vi "STED Control V2.vi"() -> ()   [LabVIEW 2014]
uses:
  FPGA-7842R-Reference.ctl
  Scan Parameters.ctl
  Manual Controls V2.ctl
  <vilib>/Utility/miscctls.llb/LVRectTypeDef.ctl
  <vilib>/Utility/miscctls.llb/LVPositionTypeDef.ctl
  Laser Controls.ctl
  XY_Stage/StageStates.ctl
  Type Defs/Image Acquisition Parameters.ctl
  Detectors.ctl
  Stage Control.ctl
panel:
  in  "Stage Control":T1={"Halt"=FALSE, "Home"=FALSE, "Down Stage"=FALSE, "Right Stage"=FALSE, "Up Stage"=FALSE, "Left Stage"=FALSE, "Mode"=enum."Joystick", "X Position"=1.0, "Y Position"=1.0, "Step Size (um)"=enum."2", "Velocity"=enum."Low"} {"Y Position" min=1.0 max=24.0}
  in  "Autoscale Z":bool
  in  "Reset Zoom":bool
  in  "Zoom Out":bool
  in  "Zoom In":bool
  in  "Pan":bool
  in  "Remove Display":bool
  in  "Add Display":bool
  in  "Colormap 2":u16(ring) items=["Fire", "Gray", "Red", "Green", "Blue", "Cyan", "Magenta", "Yellow", "Red-White", "Green-White", "Blue-White", "Glow"]
  in  "Merge Tool":bool
  in  "Smooth Tool":bool
  out "Channel 6":sgl[][](graph)
  out "Channel 5":sgl[][](graph)
  out "Channel 4":sgl[][](graph)
  out "Channel 3":sgl[][](graph)
  out "Channel 2":sgl[][](graph)
  in  "Dual Screens":bool=TRUE
  in  "Detectors":T2
  in  "Laser Controls":T3 {"590 Power (V)" scale=0.0..3.0; "STED Power (V)" scale=0.0..5.0}
  in  "Save File Path":path
  in  "Capture":bool
  in  "show cursor":bool
  in  "Set Mode Offset":bool
  in  "Unused Axis Voltage":i16=16300
  out "Channel 1":sgl[][](graph)
  in  "Image Acquisition Parameters":T4={"Scan Type"=enum."Sample Scanning", "Scan Mode"=enum."XY", "Fast Axis Frequency (Hz)"=100.0, "Image Format"=128, "Line Accumulations"=1, "Frames Per Capture"=1, "Frames Accumulations"=1, "Image Dimension (um)"=[], "Number of Z Steps"=1, "Z Steps Size (um)"=1.0, "Pixel Size (nm)"=[]} {"Z Steps Size (um)" min=0.0; "Number of Z Steps" min=1; "Frames Accumulations" min=1; "Frames Per Capture" min=1; "Line Accumulations" min=1; "Image Format" items=["64 x 64"=64, "128 x 128"=128, "256 x 256"=256, "512 x 512"=512, "1024 x 1024"=1024, "2048 x 2048"=2048]}
  in  "Live":bool
  in  "Exit":bool
  # "XY"
  # "Z"
  # "Length"
  # "Height"
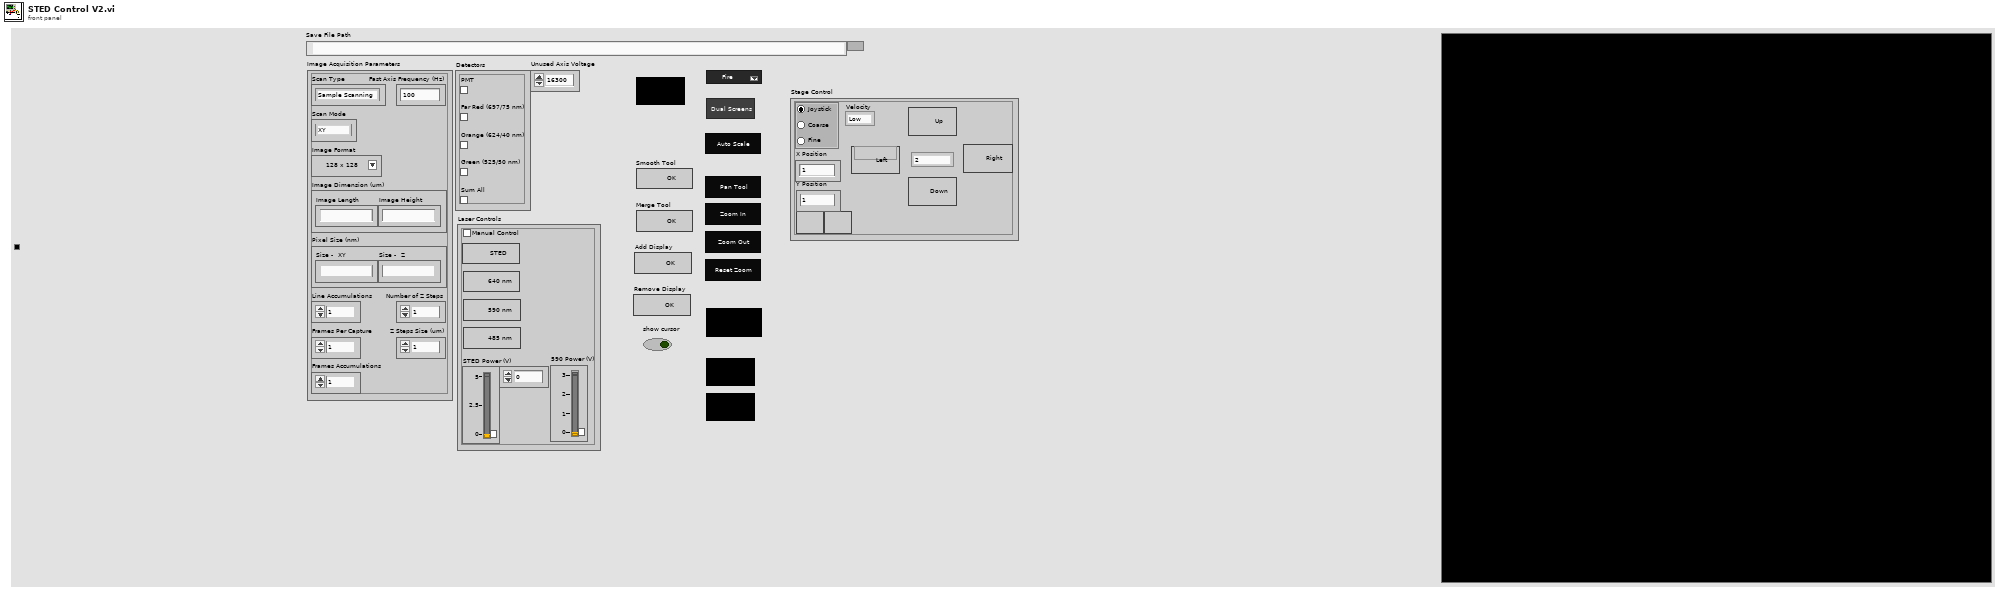
[diagram p1: front panel]
types:
  T1 = typedef "Stage Control.ctl" = cluster{"Halt":bool, "Home":bool, "Down Stage":bool, "Right Stage":bool, "Up Stage":bool, "Left Stage":bool, "Mode":enum32{"Joystick", "Coarse", "Fine"}, "X Position":dbl, "Y Position":dbl, "Step Size (um)":enum16{"1", "2", "5", "10", "15", "20", "50", "100", "500"}, "Velocity":enum16{"Low", "Medium", "High"}}
  T2 = typedef "Detectors.ctl" = cluster{"PMT":bool, "Far Red (697/75 nm)":bool, "Orange (624/40 nm)":bool, "Green (525/50 nm)":bool, "Sum All":bool}
  T3 = typedef "Laser Controls.ctl" = cluster{"STED Power (V)":dbl, "590 Power (V)":dbl, "STED":bool, "640 nm":bool, "590 nm":bool, "485 nm":bool, "Manual Control":bool}
  T4 = typedef "Image Acquisition Parameters.ctl" = cluster{"Scan Type":enum16{"Sample Scanning", "Beam Scanning"}, "Scan Mode":enum16{"XY", "XZ", "YZ", "XYZ"}, "Fast Axis Frequency (Hz)":dbl, "Image Format":u16, "Line Accumulations":u16, "Frames Per Capture":u16, "Frames Accumulations":u16, "Image Dimension (um)":dbl[], "Number of Z Steps":u8, "Z Steps Size (um)":dbl, "Pixel Size (nm)":dbl[]}
  T5 = typedef "Manual Controls V2.ctl" = cluster{"Galvo 1 Position (I16)":i16, "Galvo 2 Position (I16)":i16, "X Axis Voltage (I16)":i16, "Y Axis Voltage (I16)":i16, "Z Axis Voltage (I16)":i16, "Res Mirror Amp (I16)":i16, "Res Mirror Mute":bool}
  T6 = typedef "Scan Parameters.ctl" = cluster{"Fast_Ax_Amp_V":dbl, "Fast_Ax_Off_V":dbl, "Slow_Ax_Amp_V":dbl, "Slow_Ax_Off_V ":dbl, "Slow_Ax_Max_V_VperS":dbl, "Slow_Ax1_Del25ns":i32, "Slow_Ax2_Del25ns":i32, "Stage_X_Off_V":dbl, "Stage_Y_Off_V":dbl, "Stage_Z_Off_V":dbl, "Galvo1_Off_V":dbl, "Galvo2_Off_V":dbl, "Last_Scan_Mode":enum16{"XY", "XZ", "YZ", "XYZ"}, "Current_Scan_Mode":enum16{"XY", "XZ", "YZ", "XYZ"}, "Fly_Back_Lines":u16, "Linear_Ramp_End":u32, "Z_Step_I16":i16, "Z_Start_I16":i16, "Laser_States _U32":u32, "590_Voltage_I16":i16, "775_AOM_Volt_I16":i16, "Blanking OFF":bool, "Unused_Axis_I16":i16}
  T7 = typedef "FPGA-7842R-Reference.ctl" = enum16{"Stage Control", "Laser Control", "Unused Axis I16", "Exit", "Set Res Mirror", "Set Galvo", "Default", "Close FPGA", "Stop Waveforms", "Start Waveforms", "Initialize"}
  T8 = typedef "LVPositionTypeDef.ctl" = cluster{"Left":i32, "Top":i32}
  T9 = typedef "LVRectTypeDef.ctl" = cluster{"Left":i16, "Top":i16, "Right":i16, "Bottom":i16}
  T10 = enum32{"Invalid", "Standard", "Closed", "Hidden", "Minimized", "Maximized"}
  T11 = typedef "StageStates.ctl" = enum16{"POSITION", "MVR", "MOVE", "HALT", "ONTARGET", "ERROR", "EXIT", "HOME", "ZEROPOS", "NANOPOS", "QUIT", "SERVO", "JOYSTICK", "ANALOG"}
  T12 = typedef "LVRangeTypeDef.ctl" = cluster{"Minimum":dbl, "Maximum":dbl, "Increment":dbl, "Minor Increment":dbl, "Start":dbl}
  T13 = typedef "LVAllMonitorsDisplayTypeDef.ctl" = cluster{"Bounds":cluster{"Left":i16, "Top":i16, "Right":i16, "Bottom":i16}, "Depth":i16}[]
  T14 = cluster{"Bounds":cluster{"Left":i16, "Top":i16, "Right":i16, "Bottom":i16}, "Depth":i16}
  T15 = cluster{"Scan Type":bool, "Scan Mode":bool, "Fast Axis Frequency (Hz)":bool, "Image Format":bool, "Line Accumulations":bool, "Frames Per Capture":bool, "Frames Accumulations":bool, "Image Dimension (um)":bool[], "Number of Z Steps":bool, "Z Steps Size (um)":bool, "Pixel Size (nm)":bool[]}
  T16 = cluster{"Halt":bool, "Home":bool, "Down Stage":bool, "Right Stage":bool, "Up Stage":bool, "Left Stage":bool, "Mode":bool, "X Position":bool, "Y Position":bool, "Step Size (um)":bool, "Velocity":bool}
  T17 = enum16{"1", "2", "5", "10", "15", "20", "50", "100", "500"}
  T18 = typedef "Scanning Conversions.ctl" = cluster{"Stage X Axis (Volts/um)":dbl, "Stage Y Axis (Volts/um)":dbl, "Stage Z Axis (Volts/um)":dbl}
  T19 = typedef "IMAQ Image.ctl" = refnum<image>
  T20 = typedef "Waveform Data.ctl" = cluster{"Waveform Scan Parameters":cluster{"Scanning Mode":u8, "Fast Axis WF Length (Elements)":i32, "Fast Axis Sample Period (Ticks)":u32, "Slow Axis 1 WF Length (Elements)":i32, "Slow Axis 1 Sample Period (Ticks)":u32, "Slow Axis 1 Delay (25 ns) Steps":i32, "Slow Axis 2 WFLength (Elements)":i32, "Slow Axis 2 Sample Period (Ticks)":u32, "Slow Axis 2 Delay (25 ns) Steps":i32}, "Fast Axis Waveform":dbl[], "Slow Axis 1 Waveform":dbl[], "Slow Axis 2 Waveform":dbl[]}
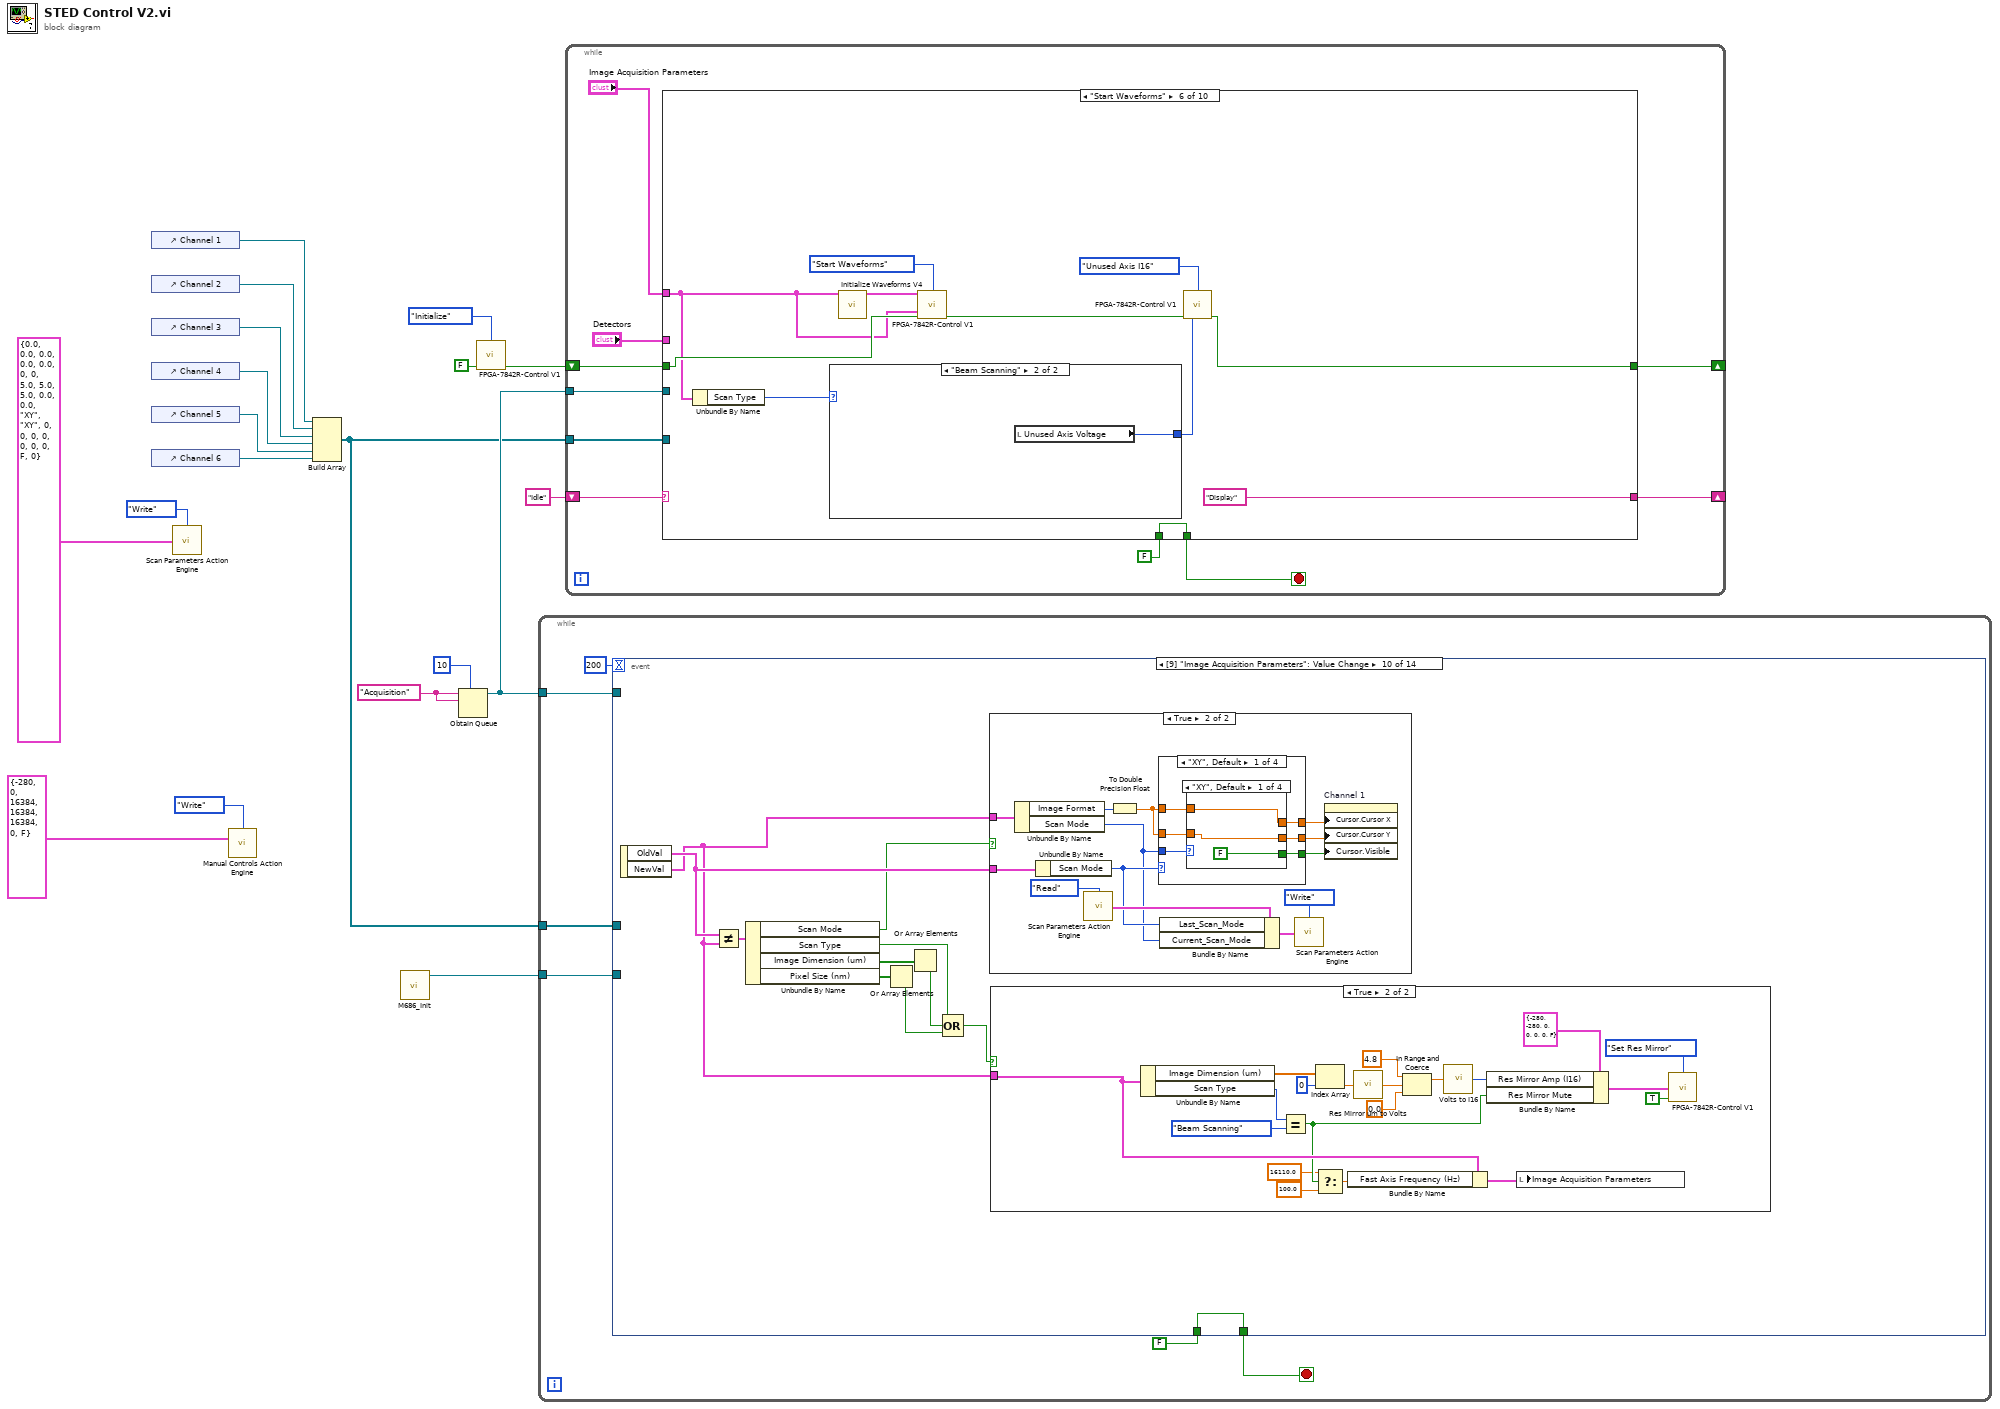
[diagram p0: block diagram]
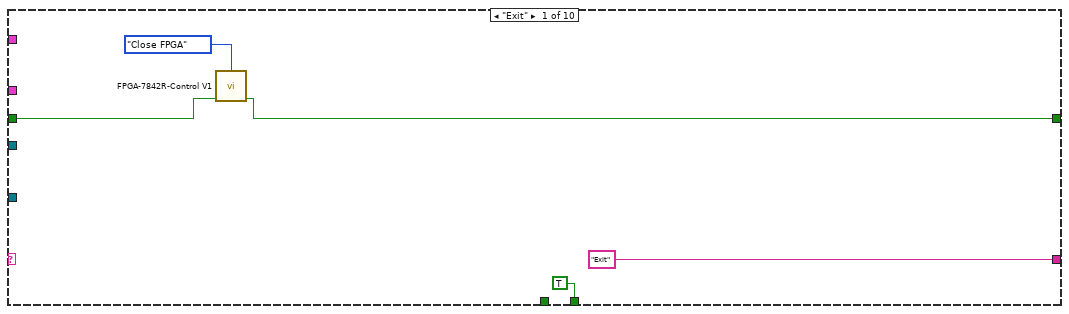
[diagram p2: hidden frame]
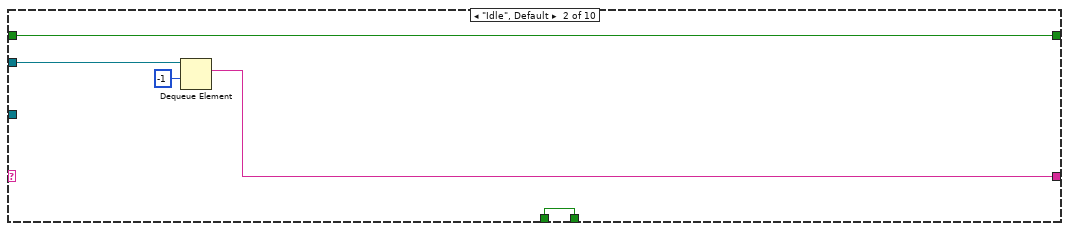
[diagram p3: hidden frame]
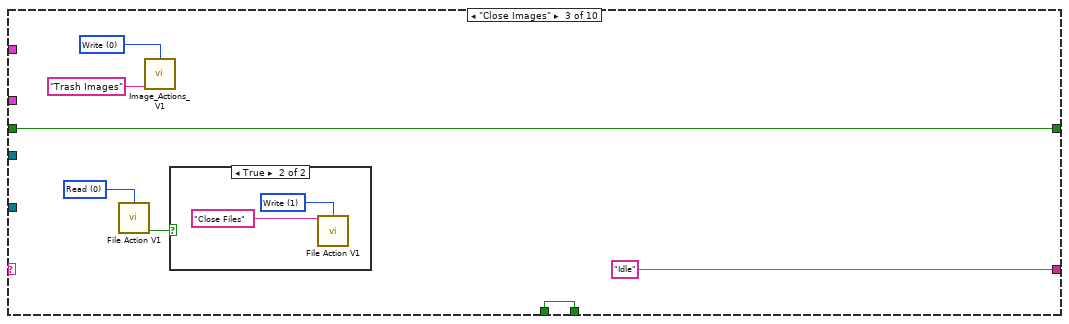
[diagram p4: hidden frame]
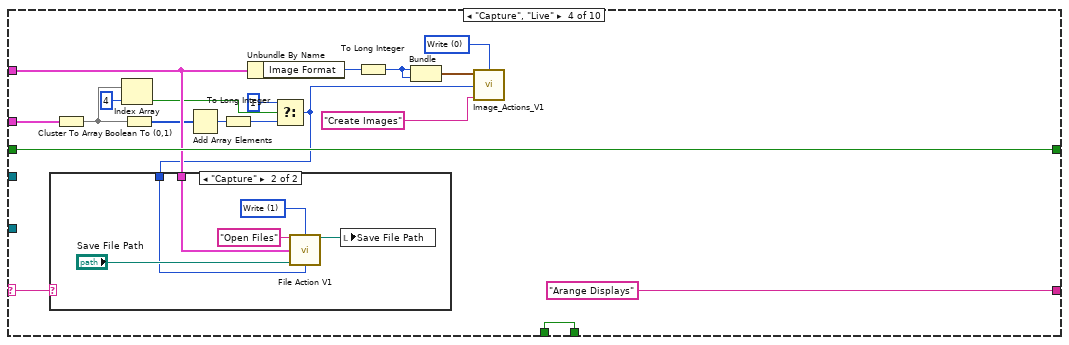
[diagram p6: hidden frame]
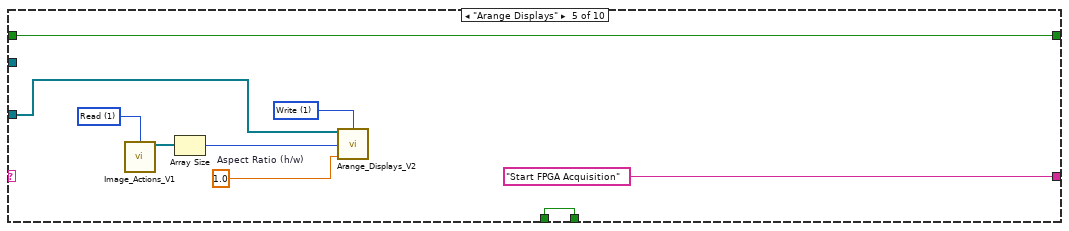
[diagram p8: hidden frame]
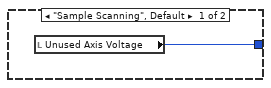
[diagram p9: hidden frame]
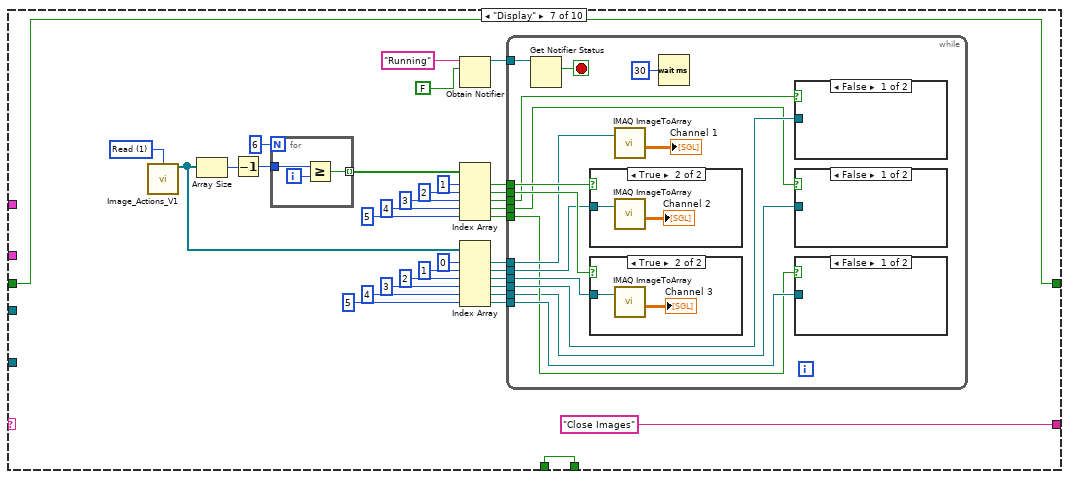
[diagram p10: hidden frame]
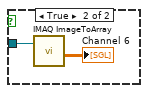
[diagram p11: hidden frame]
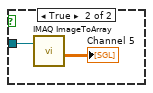
[diagram p12: hidden frame]
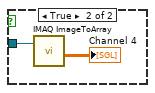
[diagram p13: hidden frame]
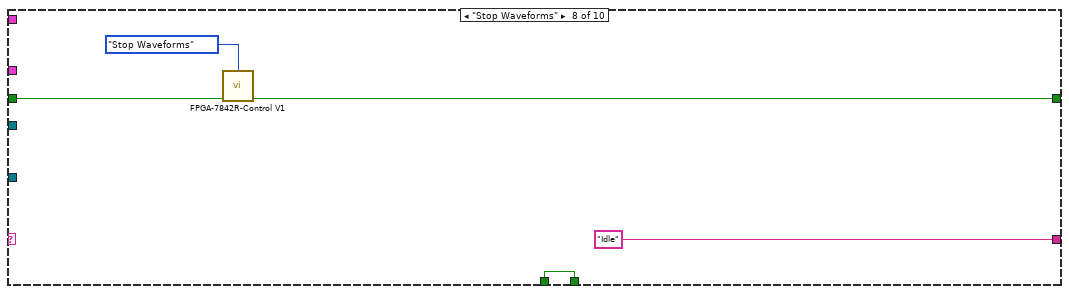
[diagram p16: hidden frame]
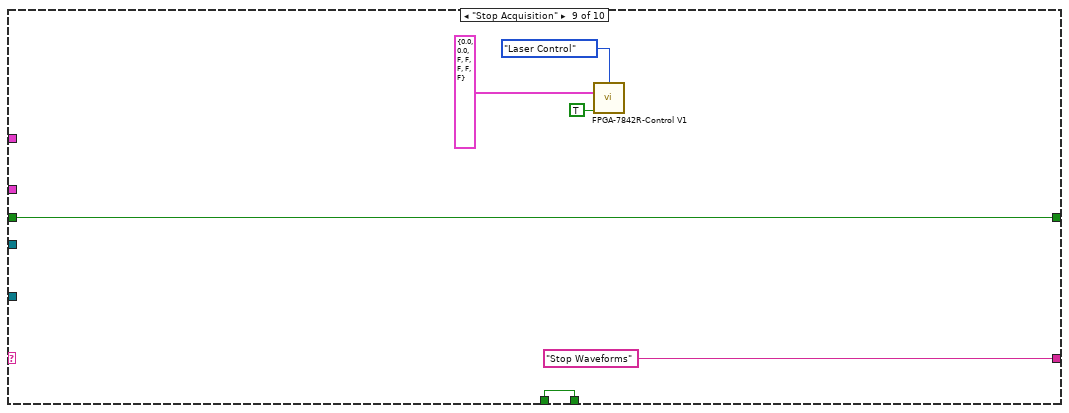
[diagram p17: hidden frame]
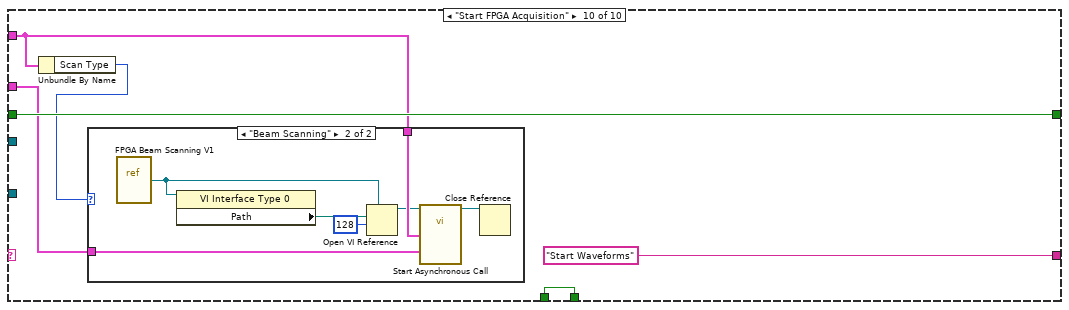
[diagram p18: hidden frame]
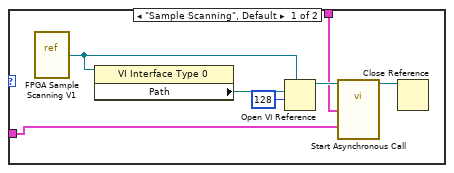
[diagram p19: hidden frame]
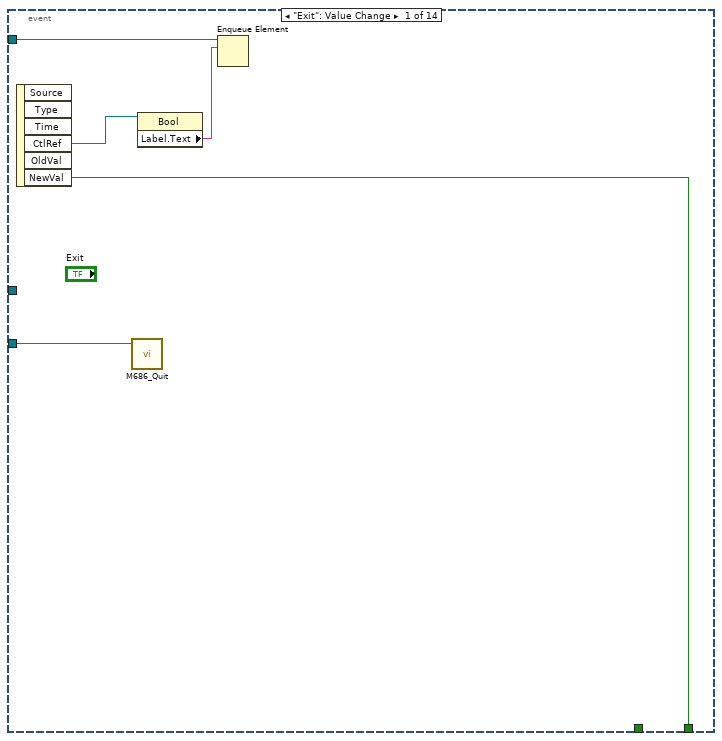
[diagram p20: hidden frame]
diagram:
  w18 = "Acquisition" ("name (unnamed)")
  n1 = control-ref of="Channel 1"() -> (w10:refnum<vi>)
  n2 = control-ref of="Channel 2"() -> (w9:refnum<vi>)
  n3 = control-ref of="Channel 3"() -> (w8:refnum<vi>)
  n4 = control-ref of="Channel 4"() -> (w7:refnum<vi>)
  n5 = control-ref of="Channel 5"() -> (w6:refnum<vi>)
  n6 = control-ref of="Channel 6"() -> (w5:refnum<vi>)
  n7 = call "Scan Parameters Action Engine.vi"("Action"=enum16{"Read", "Write"}."Write", "Scan Parameters IN"=T6 {"Fast_Ax_Amp_V"=0.0, "Fast_Ax_Off_V"=0.0, "Slow_Ax_Amp_V"=0.0, "Slow_Ax_Off_V "=0.0, "Slow_Ax_Max_V_VperS"=0.0, "Slow_Ax1_Del25ns"=0, "Slow_Ax2_Del25ns"=0, "Stage_X_Off_V"=5.0, "Stage_Y_Off_V"=5.0, "Stage_Z_Off_V"=5.0, "Galvo1_Off_V"=0.0, "Galvo2_Off_V"=0.0, "Last_Scan_Mode"=enum."XY", "Current_Scan_Mode"=enum."XY", "Fly_Back_Lines"=0, "Linear_Ramp_End"=0, "Z_Step_I16"=0, "Z_Start_I16"=0, "Laser_States _U32"=0, "590_Voltage_I16"=0, "775_AOM_Volt_I16"=0, "Blanking OFF"=FALSE, "Unused_Axis_I16"=0}) -> ()  [unwired: 13 in, 1 out]
  n8 = call "Manual Controls Action Engine.vi"("Action"=enum16{"Read", "Write"}."Write", "Manual Controls In"=T5 {"Galvo 1 Position (I16)"=-280, "Galvo 2 Position (I16)"=0, "X Axis Voltage (I16)"=16384, "Y Axis Voltage (I16)"=16384, "Z Axis Voltage (I16)"=16384, "Res Mirror Amp (I16)"=0, "Res Mirror Mute"=FALSE} ("Manual Controls")) -> ()  [unwired: 13 in, 1 out]
  n9 = Build Array(w10, w9, w8, w7, w6, w5) -> (w4:refnum<vi>[])
  n10 = call "M686_Init.vi"() -> ("VISA Refnum out"=w3:refnum<visa-resource-name>)  [unwired: 9 in, 2 out]
  n11 = Obtain Queue(max queue size (-1, unlimited)=10, name (unnamed)=w18, element data type=w18) -> (queue out=w16:refnum<queue>)  [unwired: 2 in, 2 out]
  n12 = call "FPGA-7842R-Control V1.vi"("Action"=FPGA-7842R-Reference."Initialize", "Initialize"=FALSE) -> ("Initalized"=w13:bool)  [unwired: 13 in]
  n13 = while {
    tunnel: w16 -> [w23]
    tunnel: w4 -> [w21]
    tunnel: w3 -> [w20]
    stop <- w25 stop-if-true
    n14 = event shown="[9] \"Image Acquisition Parameters\": Value Change" {
      selector: _ -> [_ _ _ _ _ _ _ _ _ _ _ _ _ _]
      dyn-events: _ -> [_ _ _ _ _ _ _ _ _ _ _ _ _ _]
      timeout: 200 -> [_ _ _ _ _ _ _ _ _ _ _ _ _ _]
      tunnel: [w30 w42 w47 w80 w107 w172 w192 w200 w227 w269 w419 w425 w611 w823] -> w25
      tunnel: FALSE -> [_ w42 w47 w80 w107 w172 w192 w200 w227 w269 w419 w425 w611 w823]
      tunnel: w23 -> [w29 w41 _ _ _ _ w186 _ _ _ _ _ _ _]
      tunnel: w21 -> [_ _ w44 _ w102 w171 _ _ _ _ _ _ _ _]
      tunnel: w20 -> [w26 _ _ _ _ _ _ _ _ _ _ w430 _ _]
      event "Exit": Value Change {
        n15 = event-data() -> ("CtlRef"=w28:refnum<vi>, "NewVal"=w30:bool)  [unwired: 1 in, 4 out]
        n16 = call "M686_Quit.vi"("VISA Refnum in"=w26) -> ()  [unwired: 11 in]
        n17 = property class="Bool"(reference=w28) -> ("Label.Text"=w27:string)  [unwired: 1 in, 2 out]
        n18 = Enqueue Element(queue=w29, element=w27) -> ()  [unwired: 2 in, 3 out]
      }
      event "Live", "Capture": Value Change {
        n19 = event-data() -> ("CtlRef"=w40:refnum<vi>, "NewVal"=w32:bool)  [unwired: 1 in]
        n20 = property on="Channel 1" class="IntGraph (strict)"("Cursor.Visible"=FALSE) -> ()  [unwired: 2 in, 2 out]
        n21 = property class="Bool (strict)"(reference=w40) -> ("Label.Text"=w31:string)  [unwired: 1 in, 2 out]
        n22 = Obtain Notifier(name (unnamed)="Running", notification data type=TRUE) -> (notifier out=w37:refnum<notifier>)  [unwired: 2 in, 2 out]
        n23 = Not(x=w32) -> (.not. x?=w35:bool)
        n24 = Send Notification(notification=w35, notifier=w37) -> ()  [unwired: 1 in, 2 out]
        n25 = Select(t=w31, s=w32, f="Stop Acquisition") -> (s? t:f=w33:string)
        n26 = Enqueue Element(queue=w41, element=w33) -> ()  [unwired: 2 in, 3 out]
      }
      event "Smooth Tool", "Merge Tool", "Add Display", "Remove Display", "Autoscale Z": Value Change {
        n27 = event-data() -> ("CtlRef"=w46:refnum<vi>)  [unwired: 1 in, 5 out]
        n28 = property class="Bool"(reference=w46) -> ("Label.Text"=w45:string)  [unwired: 1 in, 2 out]
        n29 = control-ref of="This VI"() -> (w43:refnum<vi>)
        n30 = case shown="\"Autoscale Z\"" w45 {
          tunnel: w44 -> [_ w49 w56 w61 w65 w71]
          tunnel: w43 -> [_ w48 _ _ _ w70]
          frame Default {
          }
          frame "Merge Tool" {
            n31 = vi-ref "MergeTool - Cambridge.vi"() -> (w53:refnum<vi>)
            n32 = property class="VI Interface Type 2"(reference=w53) -> ("Path"=w51:path)  [unwired: 1 in, 2 out]
            n33 = Open VI Reference(type specifier VI Refnum (for type only)=w53, vi path=w51, options=128) -> (vi reference=w52:refnum<vi>)  [unwired: 3 in, 1 out]
            n34 = call-by-ref "Start Asynchronous Call"(reference=w52, "VI Reference"=w48, "Display References"=w49) -> (reference out=w54:refnum<vi>)  [unwired: 11 in, 1 out]
            n35 = Close Reference(reference=w54) -> ()  [unwired: 1 in, 1 out]
          }
          frame "Add Display" {
            w59 = u16 1 items=["Read", "Write"] ("Action")
            w60 = u16 0 items=["Read", "Write"] ("Action")
            n36 = call "Arange_Displays_V2.vi"("Action"=w60) -> ("Number of Channels OUT"=w58:i32)  [unwired: 14 in]
            n37 = Increment(x=w58) -> (x+1=w57:i32)
            n38 = call "Arange_Displays_V2.vi"("Display References"=w56, "Action"=w59, "Number of Channels"=w57, "Aspect Ratio (h/w)"=1.0) -> ()  [unwired: 11 in, 1 out]
          }
          frame "Autoscale Z" {
            n39 = for {
              tunnel: w61 -> [w62] mode=indexing
              n40 = property class="IntGraph (strict)"(reference=w62, "ZScale.ScaleFit"=u8 1 ("Z Scale.Scale Fit")) -> ()  [unwired: 1 in, 2 out]
            }
          }
          frame "Remove Display" {
            w68 = u16 1 items=["Read", "Write"] ("Action")
            w69 = u16 0 items=["Read", "Write"] ("Action")
            n41 = call "Arange_Displays_V2.vi"("Action"=w69) -> ("Number of Channels OUT"=w67:i32)  [unwired: 14 in]
            n42 = Decrement(x=w67) -> (x-1=w66:i32)
            n43 = call "Arange_Displays_V2.vi"("Display References"=w65, "Action"=w68, "Number of Channels"=w66, "Aspect Ratio (h/w)"=1.0) -> ()  [unwired: 11 in, 1 out]
          }
          frame "Smooth Tool" {
            n44 = vi-ref "SmoothTool.vi"() -> (w73:refnum<vi>)
            n45 = property class="VI Interface Type 3"(reference=w73) -> ("Path"=w75:path)  [unwired: 1 in, 2 out]
            n46 = Open VI Reference(type specifier VI Refnum (for type only)=w73, vi path=w75, options=128) -> (vi reference=w74:refnum<vi>)  [unwired: 3 in, 1 out]
            n47 = call-by-ref "Start Asynchronous Call"(reference=w74, "VI Reference"=w70, "Display References"=w71) -> (reference out=w72:refnum<vi>)  [unwired: 2 in, 1 out]
            n48 = Close Reference(reference=w72) -> ()  [unwired: 1 in, 1 out]
          }
        }
      }
      event "Pan", "Zoom In", "Zoom Out", "Reset Zoom": Value Change {
        n49 = event-data() -> ("CtlRef"=w78:refnum<vi>, "NewVal"=w77:bool)  [unwired: 1 in]
        n50 = case shown="True" w77 {
          tunnel: w78 -> [_ w88]
          tunnel: [0 ("Palette:Active Tool") w87] -> w79
          frame False {
          }
          frame True {
            n51 = property class="Bool (strict)"(reference=w88) -> ("Label.Text"=w82:string)  [unwired: 1 in, 2 out]
            n52 = Build Array("Pan", "Zoom In", "Zoom Out") -> (w83:string[])
            n53 = case shown="\"Pan\"" w82 {
              tunnel: [6 ("Palette:Active Tool") 7 ("Palette:Active Tool") 5 ("Palette:Active Tool") 1 ("Palette:Active Tool")] -> w87
              frame "Zoom In" {
              }
              frame "Zoom Out" {
              }
              frame "Reset Zoom", Default {
              }
              frame "Pan" {
              }
            }
            n54 = for {
              tunnel: w83 -> [w89] mode=indexing
              tunnel: w82 -> [w93]
              n55 = Equal?(x=w93, y=w89) -> (x = y?=w90:bool)
              n56 = control-ref of="This VI"() -> (w91:refnum<vi>)
              n57 = To Variant(anything=w90) -> (Variant=w92:variant)
              n58 = invoke class="VI" method="Ctrl Val.Set"(reference=w91, "Control Name"=w89, "Value"=w92) -> ()  [unwired: 2 in, 5 out]
            }
          }
        }
        n59 = property on="Channel 1" class="IntGraph (strict)"("ActPaletteTool"=w79) -> ()  [unwired: 2 in, 2 out]
        n60 = property on="Channel 2" class="IntGraph (strict)"("ActPaletteTool"=w79) -> ()  [unwired: 2 in, 2 out]
        n61 = property on="Channel 3" class="IntGraph (strict)"("ActPaletteTool"=w79) -> ()  [unwired: 2 in, 2 out]
        n62 = property on="Channel 4" class="IntGraph (strict)"("ActPaletteTool"=w79) -> ()  [unwired: 2 in, 2 out]
        n63 = property on="Channel 5" class="IntGraph (strict)"("ActPaletteTool"=w79) -> ()  [unwired: 2 in, 2 out]
        n64 = property on="Channel 6" class="IntGraph (strict)"("ActPaletteTool"=w79) -> ()  [unwired: 2 in, 2 out]
      }
      event "Channel 1", "Channel 2", "Channel 3", "Channel 4", "Channel 5", "Channel 6": Mouse Down {
        n65 = event-data() -> ("CtlRef"=w103:refnum<vi>, "Mods.Double Click"=w106:bool, "PlatMods.Shift"=w105:bool, "PlatMods.Ctrl"=w104:bool)  [unwired: 1 in]
        n66 = Build Array(w106, w105, w104) -> (w99:bool[])
        n67 = property class="IntGraph (strict)"(reference=w103) -> (reference out=w101:refnum<vi>, "Label.Text"=w98:string)  [unwired: 1 in, 1 out]
        n68 = Boolean Array To Number(Boolean array=w99) -> (number=w100:u32)
        n69 = case shown="0" w100 {
          tunnel: w98 -> [w109 _ _ _ _]
          tunnel: w101 -> [_ w124 w159 w170 _]
          tunnel: w102 -> [w108 _ _ _ _]
          frame 0 {
            n70 = for {
              tunnel: w109 -> [w113]
              tunnel: w108 -> [w112] mode=indexing
              # "Single Click - Show Z Scale"
              n71 = property class="IntGraph (strict)"(reference=w112) -> (reference out=w110:refnum<vi>, "Label.Text"=w111:string)  [unwired: 1 in, 1 out]
              n72 = Equal?(x=w111, y=w113) -> (x = y?=w115:bool)
              n73 = Select(t=T8 {"Left"=2000, "Top"=17} ("Z Scale.Position"), s=w115, f=T8 {"Left"=0, "Top"=0} ("Z Scale.Position")) -> (s? t:f=w114:T8)
              n74 = property class="IntGraph (strict)"(reference=w110, "ZScale.Visible"=w115, "ZScale.Position"=w114) -> ()  [unwired: 1 in, 2 out]
            }
          }
          frame 2 {
            # "Shift Click - Apply color map."
            n75 = property class="IntGraph (strict)"(reference=w124) -> (reference out=w118:refnum<vi>, "ZScale.Maximum"=w119:dbl)  [unwired: 1 in, 1 out]
            n76 = case shown="0, Default" "Colormap 2" {
              tunnel: [cluster{dbl, u32}[] [{0.0, 0}, {85.0, 16711680}, {108.0, 16729344}, {127.0, 16744192}, {132.0, 16747520}, {140.0, 16753920}, {157.0, 16766720}, {170.0, 16776960}, {245.0, 16777184}, {250.0, 16777200}, {255.0, 16777215}] ("Z Scale.Marker Values[]") cluster{dbl, u32}[] [{0.0, 0}, {255.0, 16777215}] ("Z Scale.Marker Values[]") cluster{dbl, u32}[] [{0.0, 0}, {255.0, 16711680}] ("Z Scale.Marker Values[]") cluster{dbl, u32}[] [{0.0, 0}, {255.0, 65280}] ("Z Scale.Marker Values[]") cluster{dbl, u32}[] [{0.0, 0}, {255.0, 255}] ("Z Scale.Marker Values[]") cluster{dbl, u32}[] [{0.0, 0}, {255.0, 65535}] ("Z Scale.Marker Values[]") cluster{dbl, u32}[] [{0.0, 0}, {255.0, 16711935}] ("Z Scale.Marker Values[]") cluster{dbl, u32}[] [{0.0, 0}, {255.0, 16776960}] ("Z Scale.Marker Values[]") cluster{dbl, u32}[] [{0.0, 0}, {170.0, 16711680}, {245.0, 16777184}, {250.0, 16777200}, {255.0, 16448250}] ("Z Scale.Marker Values[]") cluster{dbl, u32}[] [{0.0, 0}, {170.0, 65280}, {245.0, 16777184}, {250.0, 16777200}, {255.0, 16448250}] ("Z Scale.Marker Values[]") cluster{dbl, u32}[] [{0.0, 0}, {170.0, 255}, {245.0, 16777184}, {250.0, 16777200}, {255.0, 16448250}] ("Z Scale.Marker Values[]") cluster{dbl, u32}[] [{0.0, 0}, {1.0, 131072}, {2.0, 196608}, {3.0, 327680}, {4.0, 458752}, {5.0, 589824}, {6.0, 720896}, {7.0, 851971}, {8.0, 983043}, {9.0, 1114115}, {10.0, 1245187}, {11.0, 1376259}, {12.0, 1507331}, {13.0, 1638403}, {14.0, 1769475}, {15.0, 1769479}, {16.0, 2031623}, {17.0, 2162695}, {18.0, 2293767}, {19.0, 2424839}, {20.0, 2555911}, {21.0, 2686983}, {22.0, 2818055}, {23.0, 2949127}, {24.0, 3080203}, {25.0, 3211275}, {26.0, 3342347}, {27.0, 3473419}, {28.0, 3604491}, {29.0, 3735563}, {30.0, 3866635}, {31.0, 3867403}, {32.0, 4129547}, {33.0, 4260619}, {34.0, 4391691}, {35.0, 4522763}, {36.0, 4653839}, {37.0, 4784911}, {38.0, 4915983}, {39.0, 5178127}, {40.0, 5309199}, {41.0, 5440271}, {42.0, 5571343}, {43.0, 5702415}, {44.0, 5703439}, {45.0, 5965583}, {46.0, 6096655}, {47.0, 6227727}, {48.0, 6358799}, {49.0, 6489871}, {50.0, 6620943}, {51.0, 6752015}, {52.0, 6883087}, {53.0, 7015183}, {54.0, 7146255}, {55.0, 7277327}, {56.0, 7408399}, {57.0, 7539471}, {58.0, 7670543}, {59.0, 7801615}, {60.0, 8063759}, {61.0, 8194831}, {62.0, 8326927}, {63.0, 8457999}, {64.0, 8589075}, {65.0, 8720147}, {66.0, 8851219}, {67.0, 8982291}, {68.0, 9113363}, {69.0, 9114387}, {70.0, 9376531}, {71.0, 9507603}, {72.0, 9638675}, {73.0, 9769747}, {74.0, 9901843}, {75.0, 10032915}, {76.0, 10163987}, {77.0, 10229523}, {78.0, 10295059}, {79.0, 10427155}, {80.0, 10558227}, {81.0, 10689299}, {82.0, 10820371}, {83.0, 10886931}, {84.0, 10952467}, {85.0, 11083539}, {86.0, 11214611}, {87.0, 11215635}, {88.0, 11477779}, {89.0, 11543315}, {90.0, 11608851}, {91.0, 11740947}, {92.0, 11806483}, {93.0, 11872019}, {94.0, 12004115}, {95.0, 12135187}, {96.0, 12266259}, {97.0, 12267283}, {98.0, 12398355}, {99.0, 12529427}, {100.0, 12530451}, {101.0, 12595987}, {102.0, 12530451}, {103.0, 12793619}, {104.0, 12794131}, {105.0, 12794643}, {106.0, 13056787}, {107.0, 13057299}, {108.0, 13057811}, {109.0, 13188883}, {110.0, 13320979}, {111.0, 13386515}, {112.0, 13452563}, {113.0, 13584147}, {114.0, 13584659}, {115.0, 13585171}, {116.0, 13585683}, {117.0, 13717267}, {118.0, 13848339}, {119.0, 13849363}, {120.0, 13849875}, {121.0, 13850387}, {122.0, 13981459}, {123.0, 14113555}, {124.0, 14114067}, {125.0, 14114579}, {126.0, 14115091}, {127.0, 14246675}, {128.0, 14377747}, {129.0, 14378771}, {130.0, 14379283}, {131.0, 14379539}, {132.0, 14379795}, {133.0, 14380819}, {134.0, 14511891}, {135.0, 14643987}, {136.0, 14644503}, {137.0, 14645015}, {138.0, 14645527}, {139.0, 14646039}, {140.0, 14646551}, {141.0, 14778135}, {142.0, 14909207}, {143.0, 14910231}, {144.0, 14910747}, {145.0, 14911259}, {146.0, 14911771}, {147.0, 14912283}, {148.0, 14912797}, {149.0, 15044383}, {150.0, 15175455}, {151.0, 15175967}, {152.0, 15176479}, {153.0, 15176991}, {154.0, 15177507}, {155.0, 15178019}, {156.0, 15178531}, {157.0, 15310115}, {158.0, 15441701}, {159.0, 15441959}, {160.0, 15442215}, {161.0, 15442727}, {162.0, 15443243}, {163.0, 15443755}, {164.0, 15444269}, {165.0, 15444783}, {166.0, 15444783}, {167.0, 15576367}, {168.0, 15707953}, {169.0, 15708467}, {170.0, 15708979}, {171.0, 15708981}, {172.0, 15708983}, {173.0, 15710011}, {174.0, 15710523}, {175.0, 15711037}, {176.0, 15711039}, {177.0, 15711553}, {178.0, 15843139}, {179.0, 15974213}, {180.0, 15974215}, {181.0, 15974217}, {182.0, 15974219}, {183.0, 15975755}, {184.0, 15976271}, {185.0, 15976785}, {186.0, 15977299}, {187.0, 15977301}, {188.0, 15977815}, {189.0, 15978327}, {190.0, 15978331}, {191.0, 16109917}, {192.0, 16241503}, {193.0, 16241505}, {194.0, 16242019}, {195.0, 16242535}, {196.0, 16242537}, {197.0, 16242539}, {198.0, 16243563}, {199.0, 16243567}, {200.0, 16244081}, {201.0, 16244595}, {202.0, 16244599}, {203.0, 16244601}, {204.0, 16244603}, {205.0, 16245627}, {206.0, 16245631}, {207.0, 16245633}, {208.0, 16246147}, {209.0, 16246663}, {210.0, 16377735}, {211.0, 16508811}, {212.0, 16508815}, {213.0, 16509839}, {214.0, 16509843}, {215.0, 16509845}, {216.0, 16509847}, {217.0, 16510361}, {218.0, 16510875}, {219.0, 16510879}, {220.0, 16510881}, {221.0, 16510883}, {222.0, 16511399}, {223.0, 16511911}, {224.0, 16511915}, {225.0, 16511917}, {226.0, 16511919}, {227.0, 16511923}, {228.0, 16512437}, {229.0, 16512951}, {230.0, 16512955}, {231.0, 16512957}, {232.0, 16512959}, {233.0, 16512961}, {234.0, 16512963}, {235.0, 16512967}, {236.0, 16513481}, {237.0, 16513995}, {238.0, 16513999}, {239.0, 16514001}, {240.0, 16514003}, {241.0, 16514005}, {242.0, 16514007}, {243.0, 16514011}, {244.0, 16514013}, {245.0, 16514015}, {246.0, 16514019}, {247.0, 16514021}, {248.0, 16514023}, {249.0, 16514027}, {250.0, 16514029}, {251.0, 16514031}, {252.0, 16514035}, {253.0, 16514037}, {254.0, 16514039}, {255.0, 16514043}] ("Z Scale.Marker Values[]")] -> w122
              tunnel: w119 -> [w125 w127 w129 w131 w133 w135 w137 w139 w141 w143 w145 w148]
              tunnel: [w125 w127 w129 w131 w133 w135 w137 w139 w141 w143 w145 w148] -> w123
              frame 0, Default {
                # "Fire"
              }
              frame 1 {
                # "Grayscale"
              }
              frame 2 {
                # "Red"
              }
              frame 3 {
                # "Green"
              }
              frame 4 {
                # "Blue"
              }
              frame 5 {
                # "Cyan"
              }
              frame 6 {
                # "Magenta"
              }
              frame 7 {
                # "Yellow"
              }
              frame 8 {
                # "Red-White"
              }
              frame 9 {
                # "Green-White"
              }
              frame 10 {
                # "Blue-White"
              }
              frame 11 {
              }
            }
            n77 = property class="IntGraph (strict)"(reference=w118, "ZScale.MarkerVals[]"=w122, "ZScale.High Color"=u32 255, "ZScale.Maximum"=w123) -> ()  [unwired: 1 in, 2 out]
          }
          frame 6 {
            w158 = u16 1 items=["Get Image", "Load and Read File"] ("Action")
            # "Shift Control Click - Open Image"
            n78 = call "OpenDBL.vi"("Action"=w158) -> ("Image"=w157:sgl[], "Dimensions (Z, Y, X, t)"=w156:i32[])  [unwired: 12 in, 1 out]
            n79 = Index Array(array=w156, index #1=1 ("index"), index #2=2 ("index")) -> (element #1=w153:i32, element #2=w151:i32)
            n80 = Reverse 1D Array(array=w157) -> (reversed array=w150:sgl[])
            n81 = Reshape Array(w150, w153, w151) -> (w152:sgl[][])
            n82 = Transpose 2D Array(2D array=w152) -> (transposed array=w149:sgl[][])
            n83 = property class="IntGraph (strict)"(reference=w159, "Value"=w149) -> ()  [unwired: 1 in, 2 out]
          }
          frame 4 {
            # "Control Click - Open for feature fitting"
            n84 = property class="IntGraph (strict)"(reference=w170) -> ("Value"=w164:sgl[][])  [unwired: 1 in, 2 out]
            n85 = local read "Image Acquisition Parameters"() -> (w163:T4)
            n86 = vi-ref "QuickProfile_V3.vi"() -> (w169:refnum<vi>)
            n87 = property class="VI Interface Type 5"(reference=w169) -> ("Path"=w166:path)  [unwired: 1 in, 2 out]
            n88 = Unbundle By Name(w163) -> ("Pixel Size (nm)"=w162:dbl[])
            n89 = Index Array(array=w162, index=0) -> (element=w160:dbl)
            n90 = Open VI Reference(type specifier VI Refnum (for type only)=w169, vi path=w166, options=128) -> (vi reference=w168:refnum<vi>)  [unwired: 3 in, 1 out]
            n91 = call-by-ref "Start Asynchronous Call"(reference=w168, "Image IN"=w164, "Pixel Size (nm)"=w160) -> (reference out=w165:refnum<vi>)  [unwired: 15 in, 1 out]
            n92 = Close Reference(reference=w165) -> ()  [unwired: 1 in, 1 out]
          }
          frame 10, Default {
            # "No match case"
          }
        }
      }
      event "Channel 1", "Channel 2", "Channel 3", "Channel 4", "Channel 5", "Channel 6": Mouse Up {
        n93 = event-data() -> ("CtlRef"=w173:refnum<vi>)  [unwired: 1 in]
        n94 = property class="IntGraph (strict)"(reference=w173) -> (reference out=w174:refnum<vi>, "ActPaletteTool"=w177:i32)  [unwired: 1 in, 1 out]
        n95 = Not Equal?(x=w177, y=0) -> (x != y?=w175:bool)
        n96 = case shown="True" w175 {
          tunnel: w174 -> [_ w181]
          tunnel: w171 -> [_ w178]
          frame False {
          }
          frame True {
            n97 = property class="IntGraph (strict)"(reference=w181) -> ("XScale.Range"=w180:T12, "YScale.Range"=w179:T12)  [unwired: 1 in, 2 out]
            n98 = for {
              tunnel: w180 -> [w183]
              tunnel: w179 -> [w184]
              tunnel: w178 -> [w182] mode=indexing
              n99 = property class="IntGraph (strict)"(reference=w182, "XScale.Range"=w183, "YScale.Range"=w184) -> ()  [unwired: 1 in, 2 out]
            }
          }
        }
      }
      event Timeout {
        n100 = event-data() -> ()  [unwired: 1 in, 3 out]
        n101 = Obtain Notifier(name (unnamed)="Running", notification data type=TRUE) -> (notifier out=w190:refnum<notifier>)  [unwired: 2 in, 2 out]
        n102 = Get Notifier Status(notifier=w190) -> (current notification=w188:bool)  [unwired: 1 in, 4 out]
        n103 = local read "Capture"() -> (w187:bool)
        n104 = And(x=w188, y=w187) -> (x .and. y?=w185:bool)
        n105 = case shown="False" w185 {
          tunnel: w186 -> [_ w194]
          frame False {
          }
          frame True {
            n106 = local write "Capture"(FALSE ("Capture")) -> ()
            n107 = Enqueue Element(queue=w194, element="Stop Acquisition" ("f")) -> ()  [unwired: 2 in, 3 out]
          }
        }
      }
      event Value Change {
        w213 = FALSE ("element")
        n108 = event-data() -> ()  [unwired: 1 in, 6 out]
        n109 = Unbundle By Name("Laser Controls") -> ("STED"=w219:bool, "640 nm"=w216:bool, "590 nm"=w217:bool, "485 nm"=w218:bool, "590 Power (V)"=w210:dbl, "STED Power (V)"=w209:dbl, "Manual Control"=w197:bool)
        n110 = Build Array(w219, w216, w217, w218, w213, w213, w213, w213) -> (w215:bool[])
        n111 = local read "Live"() -> (w198:bool)
        n112 = Boolean Array To Number(Boolean array=w215) -> (number=w214:u32)
        n113 = To Unsigned Byte Integer(number=w214) -> (unsigned 8bit integer=w212:u8)
        n114 = Or(x=w198, y=w197) -> (x .or. y?=w196:bool)
        n115 = call "U8_To_U32.vi"("U8 IN"=w212) -> ("U32 OUT"=w211:u32)  [unwired: 13 in, 1 out]
        n116 = case shown="True" w196 {
          tunnel: "Laser Controls" -> [_ w225]
          frame False {
          }
          frame True {
            n117 = call "FPGA-7842R-Control V1.vi"("Action"=FPGA-7842R-Reference."Laser Control", "Laser Controls"=w225, "Initialize"=TRUE) -> ()  [unwired: 12 in, 1 out]
          }
        }
        n118 = In Range and Coerce(upper limit=3.0, x=w210, lower limit=0.0) -> (coerced(x)=w204:dbl)  [unwired: 1 out]
        n119 = In Range and Coerce(upper limit=5.0, x=w209, lower limit=0.0) -> (coerced(x)=w203:dbl)  [unwired: 1 out]
        n120 = call "Volts to I16.vi"("Voltage (V)"=w204) -> ("I16"=w202:i16)  [unwired: 13 in, 1 out]
        n121 = call "Volts to I16.vi"("Voltage (V)"=w203) -> ("I16"=w201:i16)  [unwired: 13 in, 1 out]
        n122 = call "Scan Parameters Action Engine.vi"("Action"=enum16{"Read", "Write"}."Read") -> ("Scan Parameters OUT"=w222:T6)  [unwired: 14 in]
        n123 = Bundle By Name(cluster=w222, "Laser_States _U32"=w211, "590_Voltage_I16"=w202, "775_AOM_Volt_I16"=w201) -> (w220:T6)
        n124 = call "Scan Parameters Action Engine.vi"("Action"=enum16{"Read", "Write"}."Write", "Scan Parameters IN"=w220) -> ()  [unwired: 13 in, 1 out]
      }
      event "Dual Screens": Value Change {
        n125 = event-data() -> ("NewVal"=w229:bool)  [unwired: 1 in, 5 out]
        n126 = property class="App"() -> ("Disp.AllMonitors"=w230:T13)  [unwired: 2 in, 2 out]
        n127 = control-ref of="This VI"() -> (w228:refnum<vi>)
        n128 = case shown="False" w229 {
          tunnel: w230 -> [w233 w246]
          tunnel: T9 {"Left"=0, "Top"=0, "Right"=0, "Bottom"=0} ("FP Window Bounds 2") -> [w232 w245]
          tunnel: w228 -> [_ w244]
          frame False {
            w236 = i16 0
            n129 = Index Array(array=w233, index=0) -> (element=w240:T14)
            n130 = Unbundle By Name(w240) -> ("Bounds.Right"=w241:i16, "Bounds.Bottom"=w238:i16, "Bounds.Top"=w237:i16)
            n131 = Subtract(x=w238, y=w237) -> (x-y=w235:i16)
            n132 = Bundle By Name(cluster=w232, "Left"=w236, "Top"=w236, "Right"=w241, "Bottom"=w235) -> (w234:T9)
            n133 = property class="VI"("Front Panel.WinBounds"=w234) -> (reference out=w243:refnum<vi>)  [unwired: 2 in, 1 out]
            n134 = property class="VI"(reference=w243, "FP.State"=T10."Maximized" ("Front Panel Window:State")) -> ()  [unwired: 1 in, 2 out]
          }
          frame True {
            w255 = i16 0
            n135 = Index Array(array=w246, index #1=1 ("index"), index #2=0 ("index")) -> (element #1=w249:T14, element #2=w250:T14)
            n136 = Unbundle By Name(w249) -> ("Bounds.Right"=w251:i16)
            n137 = Unbundle By Name(w250) -> ("Bounds.Left"=w252:i16, "Bounds.Bottom"=w253:i16, "Bounds.Top"=w254:i16)
            n138 = Subtract(x=w251, y=w252) -> (x-y=w256:i16)
            n139 = Subtract(x=w253, y=w254) -> (x-y=w257:i16)
            n140 = Bundle By Name(cluster=w245, "Left"=w255, "Top"=w255, "Right"=w256, "Bottom"=w257) -> (w258:T9)
            n141 = property class="VI"(reference=w244, "Front Panel.WinBounds"=w258) -> ()  [unwired: 1 in, 2 out]
          }
        }
      }
      event Value Change {
        n142 = event-data() -> ("OldVal"=w268:T4, "NewVal"=w265:T4)  [unwired: 1 in]
        n143 = Not Equal?(x=w268, y=w265) -> (x != y?=w267:T15)
        n144 = Unbundle By Name(w267) -> ("Scan Mode"=w266:bool, "Scan Type"=w264:bool, "Image Dimension (um)"=w263:bool[], "Pixel Size (nm)"=w262:bool[])
        n145 = Or Array Elements(Boolean array=w262) -> (logical OR=w259:bool)
        n146 = Or Array Elements(Boolean array=w263) -> (logical OR=w260:bool)
        n147 = Compound Arithmetic op=OR(w264, w260, w259) -> (w261:bool)
        n148 = case shown="True" w266 {
          tunnel: w265 -> [_ w292]
          tunnel: w268 -> [_ w302]
          frame False {
            n149 = property on="Channel 1" class="IntGraph (strict)"("Cursor.Visible"=FALSE) -> ()  [unwired: 2 in, 2 out]
          }
          frame True {
            n150 = Unbundle By Name(w292) -> ("Image Format"=w303:u16, "Scan Mode"=w295:enum16{"XY", "XZ", "YZ", "XYZ"})
            n151 = Unbundle By Name(w302) -> ("Scan Mode"=w296:enum16{"XY", "XZ", "YZ", "XYZ"})
            n152 = call "Scan Parameters Action Engine.vi"("Action"=enum16{"Read", "Write"}."Read") -> ("Scan Parameters OUT"=w298:T6)  [unwired: 14 in]
            n153 = To Double Precision Float(number=w303) -> (double precision float=w291:dbl)
            n154 = case shown="\"XY\", Default" w296 {
              tunnel: w291 -> [w308 w336 w364 w392]
              tunnel: w291 -> [w307 w335 w363 w391]
              tunnel: w295 -> [w309 w337 w365 w393]
              tunnel: [w306 w334 w362 w390] -> w301
              tunnel: [w305 w333 w361 w389] -> w300
              tunnel: [w304 w332 w360 w388] -> w299
              frame "XY", Default {
                n155 = case shown="\"XY\", Default" w309 {
                  tunnel: w308 -> [w311 w318 w323 w325]
                  tunnel: w307 -> [w312 w315 w322 w329]
                  tunnel: [w311 w314 w320 w326] -> w306
                  tunnel: [w312 w313 w319 w330] -> w305
                  tunnel: [FALSE ("Cursor.Visible") TRUE ("Cursor.Visible") TRUE ("Cursor.Visible") FALSE ("Cursor.Visible")] -> w304
                  frame "XY", Default {
                  }
                  frame "XZ" {
                    n156 = Divide(x=w318, y=2.0) -> (x/y=w313:dbl)
                    n157 = Increment(x=w315) -> (x+1=w314:dbl)
                  }
                  frame "YZ" {
                    n158 = Increment(x=w323) -> (x+1=w319:dbl)
                    n159 = Divide(x=w322, y=2.0) -> (x/y=w320:dbl)
                  }
                  frame "XYZ" {
                    n160 = Divide(x=w325, y=2.0) -> (x/y=w326:dbl)
                    n161 = Divide(x=w329, y=2.0) -> (x/y=w330:dbl)
                  }
                }
              }
              frame "XZ" {
                n162 = case shown="\"XY\"" w337 {
                  tunnel: w336 -> [w339 w346 w350 w353]
                  tunnel: w335 -> [w341 w345 w348 w357]
                  tunnel: [w338 w346 w347 w354] -> w334
                  tunnel: [w340 w345 w349 w358] -> w333
                  tunnel: [TRUE ("Cursor.Visible") FALSE ("Cursor.Visible") TRUE ("Cursor.Visible") FALSE ("Cursor.Visible")] -> w332
                  frame "XY" {
                    n163 = Increment(x=w339) -> (x+1=w338:dbl)
                    n164 = Divide(x=w341, y=2.0) -> (x/y=w340:dbl)
                  }
                  frame "XZ", Default {
                  }
                  frame "YZ" {
                    n165 = Divide(x=w350, y=2.0) -> (x/y=w347:dbl)
                    n166 = Increment(x=w348) -> (x+1=w349:dbl)
                  }
                  frame "XYZ" {
                    n167 = Divide(x=w353, y=2.0) -> (x/y=w354:dbl)
                    n168 = Divide(x=w357, y=2.0) -> (x/y=w358:dbl)
                  }
                }
              }
              frame "YZ" {
                n169 = case shown="\"XYZ\"" w365 {
                  tunnel: w364 -> [w367 w375 w378 w386]
                  tunnel: w363 -> [w369 w373 w382 w387]
                  tunnel: [w366 w372 w379 w386] -> w362
                  tunnel: [w368 w374 w383 w387] -> w361
                  tunnel: [TRUE ("Cursor.Visible") TRUE ("Cursor.Visible") FALSE ("Cursor.Visible") FALSE ("Cursor.Visible")] -> w360
                  frame "XY" {
                    n170 = Increment(x=w367) -> (x+1=w366:dbl)
                    n171 = Divide(x=w369, y=2.0) -> (x/y=w368:dbl)
                  }
                  frame "XZ" {
                    n172 = Divide(x=w375, y=2.0) -> (x/y=w372:dbl)
                    n173 = Increment(x=w373) -> (x+1=w374:dbl)
                  }
                  frame "XYZ" {
                    n174 = Divide(x=w378, y=2.0) -> (x/y=w379:dbl)
                    n175 = Divide(x=w382, y=2.0) -> (x/y=w383:dbl)
                  }
                  frame "YZ", Default {
                  }
                }
              }
              frame "XYZ" {
                n176 = case shown="\"YZ\"" w393 {
                  tunnel: w392 -> [w394 w406 w411 w414]
                  tunnel: w391 -> [w398 w401 w408 w415]
                  tunnel: [w395 w405 w410 w414] -> w390
                  tunnel: [w399 w402 w409 w415] -> w389
                  tunnel: [FALSE ("Cursor.Visible") TRUE ("Cursor.Visible") TRUE ("Cursor.Visible") FALSE ("Cursor.Visible")] -> w388
                  frame "XY" {
                    n177 = Divide(x=w394, y=2.0) -> (x/y=w395:dbl)
                    n178 = Divide(x=w398, y=2.0) -> (x/y=w399:dbl)
                  }
                  frame "XZ" {
                    n179 = Divide(x=w406, y=2.0) -> (x/y=w405:dbl)
                    n180 = Increment(x=w401) -> (x+1=w402:dbl)
                  }
                  frame "YZ" {
                    n181 = Increment(x=w411) -> (x+1=w410:dbl)
                    n182 = Divide(x=w408, y=2.0) -> (x/y=w409:dbl)
                  }
                  frame "XYZ", Default {
                  }
                }
              }
            }
            n183 = Bundle By Name(cluster=w298, "Last_Scan_Mode"=w296, "Current_Scan_Mode"=w295) -> (w293:T6)
            n184 = call "Scan Parameters Action Engine.vi"("Action"=enum16{"Read", "Write"}."Write", "Scan Parameters IN"=w293) -> ()  [unwired: 13 in, 1 out]
            n185 = property on="Channel 1" class="IntGraph (strict)"("Cursor.Cursor X"=w301, "Cursor.Cursor Y"=w300, "Cursor.Visible"=w299) -> ()  [unwired: 2 in, 2 out]
          }
        }
        n186 = case shown="True" w261 {
          tunnel: w265 -> [_ w275]
          frame False {
          }
          frame True {
            n187 = Unbundle By Name(w275) -> ("Image Dimension (um)"=w289:dbl[], "Scan Type"=w284:enum16{"Sample Scanning", "Beam Scanning"})
            n188 = Equal?(x=w284, y=enum16{"Sample Scanning", "Beam Scanning"}."Beam Scanning") -> (x = y?=w274:bool)
            n189 = Index Array(array=w289, index=0) -> (element=w282:dbl)
            n190 = Select(t=16110.0, s=w274, f=100.0) -> (s? t:f=w271:dbl)
            n191 = Bundle By Name(cluster=w275, "Fast Axis Frequency (Hz)"=w271) -> (w270:T4)
            n192 = call "Res Mirror um to Volts.vi"("Image Size (um)"=w282) -> ("Voltage (V)"=w281:dbl)
            n193 = In Range and Coerce(upper limit=4.8, x=w281, lower limit=0.0) -> (coerced(x)=w280:dbl)  [unwired: 1 out]
            n194 = call "Volts to I16.vi"("Voltage (V)"=w280) -> ("I16"=w285:i16)  [unwired: 13 in, 1 out]
            n195 = Bundle By Name(cluster=T5 {"Galvo 1 Position (I16)"=-280, "Galvo 2 Position (I16)"=-280, "X Axis Voltage (I16)"=0, "Y Axis Voltage (I16)"=0, "Z Axis Voltage (I16)"=0, "Res Mirror Amp (I16)"=0, "Res Mirror Mute"=FALSE} ("Manual Controls"), "Res Mirror Amp (I16)"=w285, "Res Mirror Mute"=w274) -> (w276:T5)
            n196 = local write "Image Acquisition Parameters"(w270) -> ()
            n197 = call "FPGA-7842R-Control V1.vi"("Action"=FPGA-7842R-Reference."Set Res Mirror", "Manual Controls"=w276, "Initialize"=TRUE) -> ()  [unwired: 12 in, 1 out]
          }
        }
      }
      event "Unused Axis Voltage": Value Change {
        n198 = event-data() -> ()  [unwired: 1 in, 6 out]
        n199 = call "FPGA-7842R-Control V1.vi"("Action"=FPGA-7842R-Reference."Unused Axis I16", "Initialize"=TRUE, "Unused Axis Offset (I16)"="Unused Axis Voltage") -> ()  [unwired: 12 in, 1 out]
      }
      event Value Change {
        n200 = event-data() -> ("OldVal"=w436:T1, "NewVal"=w429:T1)  [unwired: 1 in, 4 out]
        n201 = Not Equal?(x=w436, y=w429) -> (x != y?=w435:T16)
        n202 = property on="Stage Control" class="Clust"() -> ("Controls[]"=w434:refnum<vi>[])  [unwired: 2 in, 2 out]
        n203 = Cluster To Array(cluster=w435) -> (array=w433:bool[])
        n204 = for {
          tunnel: w434 -> [w608] mode=indexing
          tunnel: w433 -> [w609] mode=indexing
          tunnel: [w608] -> w432
          stop <- w609 stop-if-true
        }
        n205 = Unbundle By Name(w429) -> ("Step Size (um)"=w426:T17, "Mode"=w431:enum32{"Joystick", "Coarse", "Fine"})
        n206 = property class="Ctl"(reference=w432) -> ("ClassName"=w428:string, "Label.Text"=w427:string)  [unwired: 1 in, 2 out]
        n207 = control-ref of="Halt"() -> (w420:refnum<vi>)
        n208 = case shown="\"Fine\"" w431 {
          tunnel: w430 -> [w443 w455 w527 w538]
          tunnel: w428 -> [_ w454 _ w537]
          tunnel: w427 -> [_ w453 _ w536]
          tunnel: w426 -> [_ w447 _ w533]
          tunnel: "Stage Control" -> [_ _ _ _]
          tunnel: [w438 w446 w526 w530] -> w423
          tunnel: w420 -> [w437 w445 w525 w529]
          frame "Joystick" {
            w442 = TRUE
            n209 = Build Array(w442, w442) -> (w441:bool[])
            n210 = call "M686.vi"("Abort"=w437, "Axis"=w441, "Action"=StageStates."JOYSTICK", "VISA In"=w443) -> ("VISA Out"=w440:refnum<visa-resource-name>)  [unwired: 4 in, 3 out]
            n211 = call "M686.vi"("Abort"=w437, "Action"=StageStates."POSITION", "VISA In"=w440) -> ("Position Out"=w438:dbl[])  [unwired: 5 in, 3 out]
          }
          frame "Coarse" {
            w457 = FALSE
            n212 = Build Array(w457, w457) -> (w456:bool[])
            n213 = Format Into String(w447) -> (resulting string=w451:string)  [unwired: 3 in, 1 out]
            n214 = call "M686.vi"("Abort"=w445, "Axis"=w456, "Action"=StageStates."JOYSTICK", "VISA In"=w455) -> ("VISA Out"=w452:refnum<visa-resource-name>)  [unwired: 4 in, 3 out]
            n215 = Fract/Exp String To Number(string=w451) -> (number=w450:dbl)  [unwired: 3 in, 1 out]
            n216 = Divide(x=w450, y=1000.0) -> (x/y=w449:dbl)
            n217 = case shown="\"Boolean\"" w454 {
              tunnel: w453 -> [_ w467]
              tunnel: w452 -> [w462 w466]
              tunnel: w449 -> [_ w465]
              tunnel: w445 -> [w459 w464]
              tunnel: [w461 w463] -> w446
              frame Default {
                n218 = call "M686.vi"("Abort"=w459, "Action"=StageStates."POSITION", "VISA In"=w462) -> ("Position Out"=w461:dbl[])  [unwired: 5 in, 3 out]
              }
              frame "Boolean" {
                n219 = case shown="\"Right\"" w467 {
                  tunnel: w466 -> [_ w472 w479 w492 w503 w514 w524]
                  tunnel: w465 -> [_ _ _ w489 w500 w511 w517]
                  tunnel: w464 -> [_ w470 w477 w484 w494 w505 w516]
                  tunnel: [dbl[] [] ("Position Out") w469 w476 w483 w493 w504 w515] -> w463
                  frame Default {
                  }
                  frame "Home" {
                    w474 = TRUE
                    n220 = Build Array(w474, w474) -> (w475:bool[])
                    n221 = call "M686.vi"("Velocity"=1.0, "Abort"=w470, "Axis"=w475, "Action"=StageStates."HOME", "VISA In"=w472) -> ("Position Out"=w469:dbl[])  [unwired: 3 in, 3 out]
                  }
                  frame "Halt" {
                    w481 = TRUE
                    n222 = Build Array(w481, w481) -> (w482:bool[])
                    n223 = call "M686.vi"("Velocity"=1.0, "Abort"=w477, "Axis"=w482, "Action"=StageStates."HALT", "VISA In"=w479) -> ("Position Out"=w476:dbl[])  [unwired: 3 in, 3 out]
                  }
                  frame "Up" {
                    n224 = Build Array(w489, w489) -> (w488:dbl[])
                    n225 = Build Array(FALSE, TRUE) -> (w485:bool[])
                    n226 = call "M686.vi"("Velocity"=1.0, "Abort"=w484, "Axis"=w485, "Positions"=w488, "Action"=StageStates."MVR", "VISA In"=w492) -> ("Position Out"=w483:dbl[])  [unwired: 2 in, 3 out]
                  }
                  frame "Down" {
                    n227 = Negate(x=w500) -> (-x=w495:dbl)
                    n228 = Build Array(w495, w495) -> (w499:dbl[])
                    n229 = Build Array(FALSE, TRUE) -> (w496:bool[])
                    n230 = call "M686.vi"("Velocity"=1.0, "Abort"=w494, "Axis"=w496, "Positions"=w499, "Action"=StageStates."MVR", "VISA In"=w503) -> ("Position Out"=w493:dbl[])  [unwired: 2 in, 3 out]
                  }
                  frame "Left" {
                    n231 = Negate(x=w511) -> (-x=w506:dbl)
                    n232 = Build Array(w506, w506) -> (w510:dbl[])
                    n233 = Build Array(TRUE, FALSE) -> (w507:bool[])
                    n234 = call "M686.vi"("Velocity"=1.0, "Abort"=w505, "Axis"=w507, "Positions"=w510, "Action"=StageStates."MVR", "VISA In"=w514) -> ("Position Out"=w504:dbl[])  [unwired: 2 in, 3 out]
                  }
                  frame "Right" {
                    n235 = Build Array(w517, w517) -> (w521:dbl[])
                    n236 = Build Array(TRUE, FALSE) -> (w518:bool[])
                    n237 = call "M686.vi"("Velocity"=1.0, "Abort"=w516, "Axis"=w518, "Positions"=w521, "Action"=StageStates."MVR", "VISA In"=w524) -> ("Position Out"=w515:dbl[])  [unwired: 2 in, 3 out]
                  }
                }
              }
            }
          }
          frame Default {
            n238 = call "M686.vi"("Abort"=w525, "Action"=StageStates."POSITION", "VISA In"=w527) -> ("Position Out"=w526:dbl[])  [unwired: 5 in, 3 out]
          }
          frame "Fine" {
            w540 = FALSE
            n239 = Build Array(w540, w540) -> (w539:bool[])
            n240 = call "M686.vi"("Abort"=w529, "Axis"=w539, "Action"=StageStates."JOYSTICK", "VISA In"=w538) -> ("VISA Out"=w532:refnum<visa-resource-name>)  [unwired: 4 in, 3 out]
            n241 = Format Into String(w533) -> (resulting string=w535:string)  [unwired: 3 in, 1 out]
            n242 = call "M686.vi"("Abort"=w529, "Action"=StageStates."POSITION", "VISA In"=w532) -> ("Position Out"=w530:dbl[])  [unwired: 5 in, 3 out]
            n243 = Fract/Exp String To Number(string=w535) -> (number=w534:dbl)  [unwired: 3 in, 1 out]
            n244 = case shown="\"Boolean\"" w537 {
              tunnel: w536 -> [_ w555]
              tunnel: w534 -> [_ w554]
              frame "False", Default {
              }
              frame "Boolean" {
                n245 = call "Manual Controls Action Engine.vi"("Action"=enum16{"Read", "Write"}."Read") -> ("Manual Controls Out"=w547:T5)  [unwired: 14 in]
                n246 = call "Scan Parameters Action Engine.vi"("Action"=enum16{"Read", "Write"}."Read") -> ("Scan Parameters OUT"=w551:T6)  [unwired: 14 in]
                n247 = call "Scanning Volts to Microns.vi"() -> ("Scanning Conversions OUT"=w553:T18)
                n248 = case shown="\"Down\"" w555 {
                  tunnel: w554 -> [_ w566 _ w583 w594 w605]
                  tunnel: w553 -> [_ w568 _ w585 w596 w607]
                  tunnel: w551 -> [w557 w563 w574 w580 w591 w602]
                  tunnel: [w557 w562 w573 w579 w590 w601] -> w549
                  tunnel: w547 -> [w556 w560 w572 w577 w588 w599]
                  tunnel: [w556 w558 w571 w575 w586 w597] -> w545
                  frame Default {
                  }
                  frame "Up" {
                    n249 = Unbundle By Name(w568) -> ("Stage Y Axis (Volts/um)"=w567:dbl)
                    n250 = Unbundle By Name(w563) -> ("Stage_Y_Off_V"=w565:dbl)
                    n251 = Multiply(x=w566, y=w567) -> (x*y=w564:dbl)
                    n252 = Add(x=w565, y=w564) -> (x+y=w561:dbl)
                    n253 = call "Volts to I16.vi"("Voltage (V)"=w561) -> ("I16"=w559:i16)  [unwired: 13 in, 1 out]
                    n254 = Bundle By Name(cluster=w563, "Stage_Y_Off_V"=w561) -> (w562:T6)
                    n255 = Bundle By Name(cluster=w560, "Y Axis Voltage (I16)"=w559) -> (w558:T5)
                  }
                  frame "Home" {
                    w570 = 5.0 ("Stage Y Axis Offset (V)")
                    n256 = call "Volts to I16.vi"("Voltage (V)"=w570) -> ("I16"=w569:i16)  [unwired: 13 in, 1 out]
                    n257 = Bundle By Name(cluster=w574, "Stage_X_Off_V"=w570, "Stage_Y_Off_V"=w570, "Stage_Z_Off_V"=w570) -> (w573:T6)
                    n258 = Bundle By Name(cluster=w572, "X Axis Voltage (I16)"=w569, "Y Axis Voltage (I16)"=w569, "Z Axis Voltage (I16)"=w569) -> (w571:T5)
                  }
                  frame "Down" {
                    n259 = Unbundle By Name(w585) -> ("Stage Y Axis (Volts/um)"=w584:dbl)
                    n260 = Unbundle By Name(w580) -> ("Stage_Y_Off_V"=w582:dbl)
                    n261 = Multiply(x=w583, y=w584) -> (x*y=w581:dbl)
                    n262 = Subtract(x=w582, y=w581) -> (x-y=w578:dbl)
                    n263 = call "Volts to I16.vi"("Voltage (V)"=w578) -> ("I16"=w576:i16)  [unwired: 13 in, 1 out]
                    n264 = Bundle By Name(cluster=w580, "Stage_Y_Off_V"=w578) -> (w579:T6)
                    n265 = Bundle By Name(cluster=w577, "Y Axis Voltage (I16)"=w576) -> (w575:T5)
                  }
                  frame "Left" {
                    n266 = Unbundle By Name(w596) -> ("Stage X Axis (Volts/um)"=w595:dbl)
                    n267 = Unbundle By Name(w591) -> ("Stage_X_Off_V"=w593:dbl)
                    n268 = Multiply(x=w594, y=w595) -> (x*y=w592:dbl)
                    n269 = Subtract(x=w593, y=w592) -> (x-y=w589:dbl)
                    n270 = call "Volts to I16.vi"("Voltage (V)"=w589) -> ("I16"=w587:i16)  [unwired: 13 in, 1 out]
                    n271 = Bundle By Name(cluster=w591, "Stage_X_Off_V"=w589) -> (w590:T6)
                    n272 = Bundle By Name(cluster=w588, "X Axis Voltage (I16)"=w587) -> (w586:T5)
                  }
                  frame "Right" {
                    n273 = Unbundle By Name(w607) -> ("Stage X Axis (Volts/um)"=w606:dbl)
                    n274 = Unbundle By Name(w602) -> ("Stage_X_Off_V"=w604:dbl)
                    n275 = Multiply(x=w605, y=w606) -> (x*y=w603:dbl)
                    n276 = Add(x=w604, y=w603) -> (x+y=w600:dbl)
                    n277 = call "Volts to I16.vi"("Voltage (V)"=w600) -> ("I16"=w598:i16)  [unwired: 13 in, 1 out]
                    n278 = Bundle By Name(cluster=w602, "Stage_X_Off_V"=w600) -> (w601:T6)
                    n279 = Bundle By Name(cluster=w599, "X Axis Voltage (I16)"=w598) -> (w597:T5)
                  }
                }
                n280 = call "Manual Controls Action Engine.vi"("Action"=enum16{"Read", "Write"}."Write", "Manual Controls In"=w545) -> ("Manual Controls Out"=w544:T5)  [unwired: 13 in]
                n281 = call "Scan Parameters Action Engine.vi"("Action"=enum16{"Read", "Write"}."Write", "Scan Parameters IN"=w549) -> ()  [unwired: 13 in, 1 out]
                n282 = call "FPGA-7842R-Control V1.vi"("Action"=FPGA-7842R-Reference."Stage Control", "Manual Controls"=w544, "Initialize"=TRUE) -> ()  [unwired: 12 in, 1 out]
              }
            }
          }
        }
        n283 = Index Array(array=w423) -> (element #1=w422:dbl, element #2=w421:dbl)  [unwired: 2 in]
        n284 = property on="X Position" class="DigNum (strict)"("Value"=w422) -> ()  [unwired: 2 in, 2 out]
        n285 = property on="Y Position" class="DigNum (strict)"("Value"=w421) -> ()  [unwired: 2 in, 2 out]
      }
      event "Set Mode Offset": Value Change {
        n286 = event-data() -> ("NewVal"=w610:bool)  [unwired: 1 in]
        n287 = case shown="True" w610 {
          frame False {
          }
          frame True {
            # "Vert Pixels"
            # "Horz Pixels"
            # "Z Pixel Size"
            # "XY Pixel Size"
            # "Z volts per um"
            # "XY volts per um"
            n288 = local read "Image Acquisition Parameters"() -> (w625:T4)
            n289 = Unbundle By Name(w625) -> ("Image Format"=w626:u16, "Image Dimension (um)"=w629:dbl[])
            n290 = call "Scanning Volts to Microns.vi"() -> ("Scanning Conversions OUT"=w614:T18)
            n291 = Unbundle By Name(w614) -> ("Stage X Axis (Volts/um)"=w613:dbl, "Stage Z Axis (Volts/um)"=w612:dbl)
            n292 = property on="Channel 1" class="IntGraph (strict)"() -> ("Cursor.Cursor X"=w620:dbl, "Cursor.Cursor Y"=w621:dbl)  [unwired: 2 in, 2 out]
            n293 = To Double Precision Float(number=w626) -> (double precision float=w617:dbl)
            n294 = call "Scan Parameters Action Engine.vi"("Action"=enum16{"Read", "Write"}."Read") -> ("Scan Parameters OUT"=w634:T6)  [unwired: 14 in]
            n295 = Divide(x=w629, y=w617) -> (x/y=w630:dbl[])
            n296 = Unbundle By Name(w634) -> ("Last_Scan_Mode"=w623:enum16{"XY", "XZ", "YZ", "XYZ"}, "Current_Scan_Mode"=w624:enum16{"XY", "XZ", "YZ", "XYZ"})
            n297 = Index Array(array=w630, index #1=0 ("index"), index #2=1 ("index")) -> (element #1=w631:dbl, element #2=w632:dbl)
            n298 = Divide(x=w617, y=2.0) -> (x/y=w616:dbl)
            n299 = case shown="\"XY\", Default" w623 {
              tunnel: w624 -> [w639 w702 w749 w796]
              tunnel: w620 -> [w640 w694 w741 w788]
              tunnel: w621 -> [w641 w695 w742 w789]
              tunnel: w616 -> [w647 w701 w748 w795]
              tunnel: w631 -> [w646 w700 w747 w794]
              tunnel: w612 -> [w644 w698 w745 w792]
              tunnel: w613 -> [w645 w699 w746 w793]
              tunnel: w632 -> [w643 w697 w744 w791]
              tunnel: w616 -> [w642 w696 w743 w790]
              tunnel: w634 -> [w638 w693 w740 w787]
              tunnel: [w637 w692 w739 w786] -> w635
              tunnel: [w636 w691 w738 w785] -> w619
              frame "XY", Default {
                # "XY Scan Mode"
                n300 = case shown="\"YZ\"" w639 {
                  tunnel: w647 -> [w656 _ w682 _]
                  tunnel: w646 -> [w658 w676 w687 _]
                  tunnel: w645 -> [w657 w674 w685 _]
                  tunnel: w644 -> [_ _ _ _]
                  tunnel: w643 -> [_ _ _ _]
                  tunnel: w642 -> [w654 w672 _ _]
                  tunnel: w641 -> [w655 w671 _ _]
                  tunnel: w640 -> [w663 _ w681 _]
                  tunnel: w638 -> [w662 w668 w680 w690]
                  tunnel: [w661 w669 w679 w690] -> w637
                  tunnel: [w666 w667 w678 w689] -> w636
                  frame "XY", Default {
                    # "XY - No change"
                    n301 = Unbundle By Name(w662) -> ("Stage_X_Off_V"=w652:dbl, "Stage_Y_Off_V"=w650:dbl, "Stage_Z_Off_V"=w666:dbl)
                    n302 = Subtract(x=w663, y=w656) -> (x-y=w665:dbl)
                    n303 = Multiply(x=w665, y=w658) -> (x*y=w664:dbl)
                    n304 = Multiply(x=w664, y=w657) -> (x*y=w653:dbl)
                    n305 = Subtract(x=w655, y=w654) -> (x-y=w659:dbl)
                    n306 = Multiply(x=w659, y=w658) -> (x*y=w660:dbl)
                    n307 = Add(x=w652, y=w653) -> (x+y=w651:dbl)
                    n308 = Multiply(x=w660, y=w657) -> (x*y=w649:dbl)
                    n309 = Add(x=w650, y=w649) -> (x+y=w648:dbl)
                    n310 = Bundle By Name(cluster=w662, "Stage_X_Off_V"=w651, "Stage_Y_Off_V"=w648) -> (w661:T6)
                  }
                  frame "XZ" {
                    # "XZ - Grab Y cusor position - Set Y offset"
                    n311 = Subtract(x=w671, y=w672) -> (x-y=w677:dbl)
                    n312 = Unbundle By Name(w668) -> ("Stage_Y_Off_V"=w670:dbl)
                    n313 = Multiply(x=w677, y=w676) -> (x*y=w675:dbl)
                    n314 = Multiply(x=w675, y=w674) -> (x*y=w673:dbl)
                    n315 = Add(x=w670, y=w673) -> (x+y=w667:dbl)
                    n316 = Bundle By Name(cluster=w668, "Stage_Y_Off_V"=w667) -> (w669:T6)
                  }
                  frame "YZ" {
                    # "YZ - Grab X cursor position - Set X offset"
                    n317 = Subtract(x=w681, y=w682) -> (x-y=w688:dbl)
                    n318 = Unbundle By Name(w680) -> ("Stage_X_Off_V"=w684:dbl)
                    n319 = Multiply(x=w688, y=w687) -> (x*y=w686:dbl)
                    n320 = Multiply(x=w686, y=w685) -> (x*y=w683:dbl)
                    n321 = Add(x=w684, y=w683) -> (x+y=w678:dbl)
                    n322 = Bundle By Name(cluster=w680, "Stage_X_Off_V"=w678) -> (w679:T6)
                  }
                  frame "XYZ" {
                    # "XYZ - No change"
                    n323 = Unbundle By Name(w690) -> ("Stage_Z_Off_V"=w689:dbl)
                  }
                }
              }
              frame "XZ" {
                # "XZ Scan Mode"
                n324 = case shown="\"YZ\"" w702 {
                  tunnel: w701 -> [_ _ w718 _]
                  tunnel: w700 -> [_ _ w725 _]
                  tunnel: w699 -> [_ _ w722 _]
                  tunnel: w698 -> [w705 _ _ w729]
                  tunnel: w693 -> [w712 w715 w724 w736]
                  tunnel: w697 -> [w704 _ _ w728]
                  tunnel: [w709 w715 w719 w733] -> w692
                  tunnel: w696 -> [w708 _ _ w732]
                  tunnel: w695 -> [w707 _ _ w731]
                  tunnel: w694 -> [_ _ w717 _]
                  tunnel: [w703 w714 w716 w727] -> w691
                  frame "XY", Default {
                    # "XY - Grab Y cusor position - Set Z offset"
                    n325 = Subtract(x=w707, y=w708) -> (x-y=w713:dbl)
                    n326 = Unbundle By Name(w712) -> ("Stage_Z_Off_V"=w706:dbl)
                    n327 = Multiply(x=w713, y=w704) -> (x*y=w711:dbl)
                    n328 = Multiply(x=w711, y=w705) -> (x*y=w710:dbl)
                    n329 = Add(x=w706, y=w710) -> (x+y=w703:dbl)
                    n330 = Bundle By Name(cluster=w712, "Stage_Z_Off_V"=w703) -> (w709:T6)
                  }
                  frame "XZ" {
                    # "XZ - No change"
                    n331 = Unbundle By Name(w715) -> ("Stage_Z_Off_V"=w714:dbl)
                  }
                  frame "YZ" {
                    # "YZ - Grab X cursor position - Set X offset"
                    n332 = Subtract(x=w717, y=w718) -> (x-y=w726:dbl)
                    n333 = Unbundle By Name(w724) -> ("Stage_X_Off_V"=w721:dbl)
                    n334 = Multiply(x=w726, y=w725) -> (x*y=w723:dbl)
                    n335 = Multiply(x=w723, y=w722) -> (x*y=w720:dbl)
                    n336 = Add(x=w721, y=w720) -> (x+y=w716:dbl)
                    n337 = Bundle By Name(cluster=w724, "Stage_X_Off_V"=w716) -> (w719:T6)
                  }
                  frame "XYZ" {
                    # "XYZ - Grab Y cusor position - Set Z offset"
                    n338 = Subtract(x=w731, y=w732) -> (x-y=w737:dbl)
                    n339 = Unbundle By Name(w736) -> ("Stage_Z_Off_V"=w730:dbl)
                    n340 = Multiply(x=w737, y=w728) -> (x*y=w735:dbl)
                    n341 = Multiply(x=w735, y=w729) -> (x*y=w734:dbl)
                    n342 = Add(x=w730, y=w734) -> (x+y=w727:dbl)
                    n343 = Bundle By Name(cluster=w736, "Stage_Z_Off_V"=w727) -> (w733:T6)
                  }
                }
              }
              frame "YZ" {
                # "YZ Scan Mode"
                n344 = case shown="\"XZ\"" w749 {
                  tunnel: w748 -> [_ w763 _ _]
                  tunnel: w747 -> [_ w770 _ _]
                  tunnel: w746 -> [_ w767 _ _]
                  tunnel: w745 -> [w752 _ _ w776]
                  tunnel: w740 -> [w759 w769 w773 w783]
                  tunnel: w744 -> [w751 _ _ w775]
                  tunnel: [w756 w764 w773 w780] -> w739
                  tunnel: w743 -> [w755 _ _ w779]
                  tunnel: w742 -> [w754 _ _ w778]
                  tunnel: w741 -> [_ w762 _ _]
                  tunnel: [w750 w761 w772 w774] -> w738
                  frame "XY", Default {
                    # "XY - Grab Y cusor position - Set Z offset"
                    n345 = Subtract(x=w754, y=w755) -> (x-y=w760:dbl)
                    n346 = Unbundle By Name(w759) -> ("Stage_Z_Off_V"=w753:dbl)
                    n347 = Multiply(x=w760, y=w751) -> (x*y=w758:dbl)
                    n348 = Multiply(x=w758, y=w752) -> (x*y=w757:dbl)
                    n349 = Add(x=w753, y=w757) -> (x+y=w750:dbl)
                    n350 = Bundle By Name(cluster=w759, "Stage_Z_Off_V"=w750) -> (w756:T6)
                  }
                  frame "XZ" {
                    # "XZ - Grab X cursor position - Set Y offset"
                    n351 = Subtract(x=w762, y=w763) -> (x-y=w771:dbl)
                    n352 = Unbundle By Name(w769) -> ("Stage_Y_Off_V"=w766:dbl)
                    n353 = Multiply(x=w771, y=w770) -> (x*y=w768:dbl)
                    n354 = Multiply(x=w768, y=w767) -> (x*y=w765:dbl)
                    n355 = Add(x=w766, y=w765) -> (x+y=w761:dbl)
                    n356 = Bundle By Name(cluster=w769, "Stage_Y_Off_V"=w761) -> (w764:T6)
                  }
                  frame "YZ" {
                    # "YZ - No change"
                    n357 = Unbundle By Name(w773) -> ("Stage_Z_Off_V"=w772:dbl)
                  }
                  frame "XYZ" {
                    # "XYZ - Grab Y cusor position - Set Z offset"
                    n358 = Subtract(x=w778, y=w779) -> (x-y=w784:dbl)
                    n359 = Unbundle By Name(w783) -> ("Stage_Z_Off_V"=w777:dbl)
                    n360 = Multiply(x=w784, y=w775) -> (x*y=w782:dbl)
                    n361 = Multiply(x=w782, y=w776) -> (x*y=w781:dbl)
                    n362 = Add(x=w777, y=w781) -> (x+y=w774:dbl)
                    n363 = Bundle By Name(cluster=w783, "Stage_Z_Off_V"=w774) -> (w780:T6)
                  }
                }
              }
              frame "XYZ" {
                # "XYZ Scan Mode"
                n364 = case shown="\"XZ\"" w796 {
                  tunnel: w795 -> [_ _ w812 _]
                  tunnel: w794 -> [_ w808 w819 _]
                  tunnel: w793 -> [_ w805 w816 _]
                  tunnel: w792 -> [_ _ _ _]
                  tunnel: w787 -> [w798 w807 w818 w822]
                  tunnel: w791 -> [_ _ _ _]
                  tunnel: [w798 w803 w813 w822] -> w786
                  tunnel: w790 -> [_ w802 _ _]
                  tunnel: w789 -> [_ w801 _ _]
                  tunnel: w788 -> [_ _ w811 _]
                  tunnel: [w797 w799 w810 w821] -> w785
                  frame "XY", Default {
                    # "XY - No change"
                    n365 = Unbundle By Name(w798) -> ("Stage_Z_Off_V"=w797:dbl)
                  }
                  frame "XZ" {
                    # "XZ - Grab Y cusor position - Set Y offset"
                    n366 = Subtract(x=w801, y=w802) -> (x-y=w809:dbl)
                    n367 = Unbundle By Name(w807) -> ("Stage_Y_Off_V"=w800:dbl)
                    n368 = Multiply(x=w809, y=w808) -> (x*y=w806:dbl)
                    n369 = Multiply(x=w806, y=w805) -> (x*y=w804:dbl)
                    n370 = Add(x=w800, y=w804) -> (x+y=w799:dbl)
                    n371 = Bundle By Name(cluster=w807, "Stage_Y_Off_V"=w799) -> (w803:T6)
                  }
                  frame "YZ" {
                    # "YZ - Grab X cursor position - Set X offset"
                    n372 = Subtract(x=w811, y=w812) -> (x-y=w820:dbl)
                    n373 = Unbundle By Name(w818) -> ("Stage_X_Off_V"=w815:dbl)
                    n374 = Multiply(x=w820, y=w819) -> (x*y=w817:dbl)
                    n375 = Multiply(x=w817, y=w816) -> (x*y=w814:dbl)
                    n376 = Add(x=w815, y=w814) -> (x+y=w810:dbl)
                    n377 = Bundle By Name(cluster=w818, "Stage_X_Off_V"=w810) -> (w813:T6)
                  }
                  frame "XYZ" {
                    # "XYZ - No change"
                    n378 = Unbundle By Name(w822) -> ("Stage_Z_Off_V"=w821:dbl)
                  }
                }
              }
            }
            n379 = call "Volts to I16.vi"("Voltage (V)"=w619) -> ("I16"=w618:i16)  [unwired: 13 in, 1 out]
            n380 = local write "Unused Axis Voltage"(w618) -> ()
            n381 = call "Scan Parameters Action Engine.vi"("Action"=enum16{"Read", "Write"}."Write", "Scan Parameters IN"=w635) -> ()  [unwired: 13 in, 1 out]
          }
        }
      }
      event "show cursor": Value Change {
        w824 = 50.0 ("Cursor.Cursor Position:Cursor X")
        n382 = event-data() -> ("NewVal"=w825:bool)  [unwired: 1 in, 5 out]
        n383 = property on="Channel 1" class="IntGraph (strict)"("Cursor.Cursor X"=w824, "Cursor.Cursor Y"=w824, "Cursor.Visible"=w825) -> ()  [unwired: 2 in, 2 out]
      }
    }
  }
  n384 = while {
    shift-right: [w834] -> _
    shift-left: "Idle" -> [w835]
    tunnel: w16 -> [w831]
    shift-right: [w829] -> _
    shift-left: w13 -> [w830]
    tunnel: w4 -> [w826]
    stop <- w833 stop-if-true
    n385 = case shown="\"Start Waveforms\"" w835 {
      selector: w835 -> [_ _ _ w865 _ _ _ _ _ _]
      tunnel: ["Exit" w842 "Idle" ("name (unnamed)") "Arange Displays" ("name (unnamed)") "Start FPGA Acquisition" ("name (unnamed)") "Display" ("name (unnamed)") "Close Images" ("name (unnamed)") "Idle" "Stop Waveforms" ("name (unnamed)") "Start Waveforms" ("name (unnamed)")] -> w834
      tunnel: [TRUE w844 w851 w873 w887 w899 w935 w968 w973 w979] -> w833
      tunnel: FALSE -> [_ w844 w851 w873 w887 w899 w935 w968 w973 w979]
      tunnel: w831 -> [_ w843 _ _ _ _ _ _ _ _]
      tunnel: w830 -> [w838 w841 w852 w871 w884 w897 w933 w966 w974 w980]
      tunnel: [w837 w841 w852 w871 w884 w892 w933 w965 w974 w980] -> w829
      tunnel: "Image Acquisition Parameters" -> [_ _ _ w864 _ w889 _ _ _ w977]
      tunnel: "Detectors" -> [_ _ _ w863 _ _ _ _ _ w975]
      tunnel: w826 -> [_ _ _ _ w880 _ _ _ _ _]
      frame "Exit" {
        n386 = call "FPGA-7842R-Control V1.vi"("Action"=FPGA-7842R-Reference."Close FPGA", "Initialize"=w838) -> ("Initalized"=w837:bool)  [unwired: 13 in]
      }
      frame "Idle", Default {
        n387 = Dequeue Element(queue=w843, timeout in ms (-1)=-1) -> (element=w842:string)  [unwired: 1 in, 3 out]
      }
      frame "Close Images" {
        w847 = u16 0 items=["Read", "Write"] ("Mode")
        w848 = u16 0 items=["Write", "Read"] ("Mode")
        n388 = call "File Action V1.vi"("Mode"=w847) -> ("Files Open"=w846:bool)  [unwired: 12 in, 2 out]
        n389 = call "Image_Actions_V1.vi"("Mode"=w848, "Action"="Trash Images") -> ()  [unwired: 12 in, 2 out]
        n390 = case shown="True" w846 {
          frame False {
          }
          frame True {
            w854 = u16 1 items=["Read", "Write"] ("Mode")
            n391 = call "File Action V1.vi"("Action"="Close Files", "Mode"=w854) -> ()  [unwired: 11 in, 3 out]
          }
        }
      }
      frame "Capture", "Live" {
        w869 = u16 0 items=["Write", "Read"] ("Mode")
        n392 = Cluster To Array(cluster=w863) -> (array=w861:bool[])
        n393 = Index Array(array=w861, index=4) -> (element=w858:bool)
        n394 = Boolean To (0,1)(Boolean=w861) -> (0, 1=w862:i16[])
        n395 = Add Array Elements(numeric array=w862) -> (sum=w859:i16)
        n396 = To Long Integer(number=w859) -> (32bit integer=w856:i32)
        n397 = Unbundle By Name(w864) -> ("Image Format"=w866:u16)
        n398 = Select(t=1, s=w858, f=w856) -> (s? t:f=w855:i32)
        n399 = case shown="\"Capture\"" w865 {
          tunnel: w864 -> [_ w875]
          tunnel: w855 -> [_ w874]
          frame Default {
          }
          frame "Capture" {
            w878 = u16 1 items=["Read", "Write"] ("Mode")
            n400 = call "File Action V1.vi"("Action"="Open Files", "Mode"=w878, "Image Acquisition Parameters"=w875, "File Path IN"="Save File Path", "Number of Channels"=w874) -> ("File Path OUT"=w876:path)  [unwired: 8 in, 2 out]
            n401 = local write "Save File Path"(w876) -> ()
          }
        }
        n402 = To Long Integer(number=w866) -> (32bit integer=w868:i32)
        n403 = Bundle(w868, w868) -> (w867:cluster{i32, i32})  [unwired: 1 in]
        n404 = call "Image_Actions_V1.vi"("Image Size (Pixels)"=w867, "Mode"=w869, "Number of Channels"=w855, "Action"="Create Images") -> ()  [unwired: 10 in, 2 out]
      }
      frame "Arange Displays" {
        w882 = u16 1 items=["Write", "Read"] ("Mode")
        w886 = 1.0  # Aspect Ratio (h/w)
        w885 = u16 1 items=["Read", "Write"] ("Action")
        n405 = call "Image_Actions_V1.vi"("Mode"=w882) -> ("Image REFs OUT"=w883:T19[])  [unwired: 13 in, 1 out]
        n406 = Array Size(array=w883) -> (size(s)=w881:i32)
        n407 = call "Arange_Displays_V2.vi"("Display References"=w880, "Action"=w885, "Number of Channels"=w881, "Aspect Ratio (h/w)"=w886) -> ()  [unwired: 11 in, 1 out]
      }
      frame "Start Waveforms" {
        n408 = Unbundle By Name(w889) -> ("Scan Type"=w891:enum16{"Sample Scanning", "Beam Scanning"})
        n409 = case shown="\"Beam Scanning\"" w891 {
          tunnel: [w900 w901] -> w890
          frame "Sample Scanning", Default {
            n410 = local read "Unused Axis Voltage"() -> (w900:i16)
          }
          frame "Beam Scanning" {
            n411 = local read "Unused Axis Voltage"() -> (w901:i16)
          }
        }
        n412 = call "Initialize Waveforms V4.vi"("Image Acquisition Parameters"=w889) -> ("Waveform Data to FPGA"=w898:T20)  [unwired: 14 in]
        n413 = call "FPGA-7842R-Control V1.vi"("Waveform Data"=w898, "Action"=FPGA-7842R-Reference."Start Waveforms", "Image Acquisition Parameters"=w889, "Initialize"=w897) -> ("Initalized"=w893:bool)  [unwired: 11 in]
        n414 = call "FPGA-7842R-Control V1.vi"("Action"=FPGA-7842R-Reference."Unused Axis I16", "Initialize"=w893, "Unused Axis Offset (I16)"=w890) -> ("Initalized"=w892:bool)  [unwired: 12 in]
      }
      frame "Display" {
        w927 = u16 1 items=["Write", "Read"] ("Mode")
        n415 = call "Image_Actions_V1.vi"("Mode"=w927) -> ("Image REFs OUT"=w929:T19[])  [unwired: 13 in, 1 out]
        n416 = Array Size(array=w929) -> (size(s)=w925:i32)
        n417 = Decrement(x=w925) -> (x-1=w924:i32)
        n418 = for {
          N: 6 -> [_]
          tunnel: w924 -> [w963]
          tunnel: [w961] -> w928 mode=indexing
          i -> [w962]
          n419 = Greater Or Equal?(x=w963, y=w962) -> (x >= y?=w961:bool)
        }
        n420 = Obtain Notifier(name (unnamed)="Running", notification data type=FALSE) -> (notifier out=w932:refnum<notifier>)  [unwired: 2 in, 2 out]
        n421 = Index Array(array=w928, index #1=1 ("index"), index #2=2 ("index"), index #3=3 ("index"), index #4=4 ("index"), index #5=5 ("index")) -> (element #1=w913:bool, element #2=w912:bool, element #3=w911:bool, element #4=w910:bool, element #5=w909:bool)
        n422 = Index Array(array=w929, index #1=0 ("index"), index #2=1 ("index"), index #3=2 ("index"), index #4=3 ("index"), index #5=4 ("index"), index #6=5 ("index")) -> (element #1=w908:T19, element #2=w907:T19, element #3=w906:T19, element #4=w905:T19, element #5=w904:T19, element #6=w903:T19)
        n423 = while {
          tunnel: w913 -> [w950]
          tunnel: w912 -> [w949]
          tunnel: w911 -> [w945]
          tunnel: w910 -> [w942]
          tunnel: w909 -> [w941]
          tunnel: w908 -> [w948]
          tunnel: w907 -> [w947]
          tunnel: w906 -> [w946]
          tunnel: w905 -> [w944]
          tunnel: w904 -> [w938]
          tunnel: w903 -> [w943]
          tunnel: w932 -> [w940]
          stop <- w939 stop-if-true
          n424 = Get Notifier Status(notifier=w940) -> (current notification=w939:bool)  [unwired: 1 in, 4 out]
          n425 = case shown="True" w950 {
            tunnel: w947 -> [_ w960]
            frame False {
            }
            frame True {
              n426 = call "IMAQ ImageToArray"("Image"=w960) -> ("Image Pixels (Float)"=→"Channel 2":sgl[][])  [unwired: 3 in, 4 out]
            }
          }
          n427 = case shown="True" w949 {
            tunnel: w946 -> [_ w958]
            frame False {
            }
            frame True {
              n428 = call "IMAQ ImageToArray"("Image"=w958) -> ("Image Pixels (Float)"=→"Channel 3":sgl[][])  [unwired: 3 in, 4 out]
            }
          }
          n429 = call "IMAQ ImageToArray"("Image"=w948) -> ("Image Pixels (Float)"=→"Channel 1":sgl[][])  [unwired: 3 in, 4 out]
          n430 = Wait (ms)(milliseconds to wait=u32 30) -> ()  [unwired: 1 out]
          n431 = case shown="False" w945 {
            tunnel: w944 -> [_ w956]
            frame False {
            }
            frame True {
              n432 = call "IMAQ ImageToArray"("Image"=w956) -> ("Image Pixels (Float)"=→"Channel 4":sgl[][])  [unwired: 3 in, 4 out]
            }
          }
          n433 = case shown="False" w942 {
            tunnel: w938 -> [_ w954]
            frame False {
            }
            frame True {
              n434 = call "IMAQ ImageToArray"("Image"=w954) -> ("Image Pixels (Float)"=→"Channel 5":sgl[][])  [unwired: 3 in, 4 out]
            }
          }
          n435 = case shown="False" w941 {
            tunnel: w943 -> [_ w952]
            frame False {
            }
            frame True {
              n436 = call "IMAQ ImageToArray"("Image"=w952) -> ("Image Pixels (Float)"=→"Channel 6":sgl[][])  [unwired: 3 in, 4 out]
            }
          }
        }
      }
      frame "Stop Waveforms" {
        n437 = call "FPGA-7842R-Control V1.vi"("Action"=FPGA-7842R-Reference."Stop Waveforms", "Initialize"=w966) -> ("Initalized"=w965:bool)  [unwired: 13 in]
      }
      frame "Stop Acquisition" {
        n438 = call "FPGA-7842R-Control V1.vi"("Action"=FPGA-7842R-Reference."Laser Control", "Laser Controls"=T3 {"STED Power (V)"=0.0, "590 Power (V)"=0.0, "STED"=FALSE, "640 nm"=FALSE, "590 nm"=FALSE, "485 nm"=FALSE, "Manual Control"=FALSE} ("Laser Controls 2"), "Initialize"=TRUE) -> ()  [unwired: 12 in, 1 out]
      }
      frame "Start FPGA Acquisition" {
        n439 = Unbundle By Name(w977) -> ("Scan Type"=w976:enum16{"Sample Scanning", "Beam Scanning"})
        n440 = case shown="\"Beam Scanning\"" w976 {
          tunnel: w977 -> [w982 w990]
          tunnel: w975 -> [w981 w988]
          frame "Sample Scanning", Default {
            n441 = vi-ref "FPGA Sample Scanning V1.vi"() -> (w985:refnum<vi>)
            n442 = property class="VI Interface Type 0"(reference=w985) -> ("Path"=w983:path)  [unwired: 1 in, 2 out]
            n443 = Open VI Reference(type specifier VI Refnum (for type only)=w985, vi path=w983, options=128) -> (vi reference=w986:refnum<vi>)  [unwired: 3 in, 1 out]
            n444 = call-by-ref "Start Asynchronous Call"(reference=w986, "Detectors"=w981, "Image Acquisition Parameters"=w982) -> (reference out=w987:refnum<vi>)  [unwired: 2 in, 1 out]
            n445 = Close Reference(reference=w987) -> ()  [unwired: 1 in, 1 out]
          }
          frame "Beam Scanning" {
            n446 = vi-ref "FPGA Beam Scanning V1.vi"() -> (w993:refnum<vi>)
            n447 = property class="VI Interface Type 0"(reference=w993) -> ("Path"=w991:path)  [unwired: 1 in, 2 out]
            n448 = Open VI Reference(type specifier VI Refnum (for type only)=w993, vi path=w991, options=128) -> (vi reference=w989:refnum<vi>)  [unwired: 3 in, 1 out]
            n449 = call-by-ref "Start Asynchronous Call"(reference=w989, "Detectors"=w988, "Image Acquisition Parameters"=w990) -> (reference out=w994:refnum<vi>)  [unwired: 2 in, 1 out]
            n450 = Close Reference(reference=w994) -> ()  [unwired: 1 in, 1 out]
          }
        }
      }
    }
  }
